vi "HiSPARC Weather Station.vi"() -> ()   [LabVIEW 2012]
uses:
  Globals/Status_Error_Messages.vi
  Globals/Re_Connection_Counter.vi
  Globals/Re_Initialisation_Counter.vi
  Globals/Stop_Data_Loop.vi
  Globals/Stop_Button_Loop.vi
  Globals/USB_WeatherLink_Serialnumber.vi
  Globals/Help_URL.vi
  Globals/DAQ_Mode.vi
  <vilib>/Utility/config.llb/Read Key (Double).vi
  <vilib>/Utility/config.llb/Read Key (Boolean).vi
  <vilib>/Utility/config.llb/Read Key (String).vi
  <vilib>/Utility/config.llb/Read Key (I32).vi
  Globals/TempHumWindDir_Calibration.vi
  Globals/Barometer_Calibration.vi
  Globals/Station_Coordinates.vi
  <vilib>/Platform/browser.llb/Open URL in Default Browser (string).vi
  <vilib>/Utility/config.llb/Write Key (I32).vi
  Globals/PCtime_Last_Data.vi
  <vilib>/Utility/config.llb/Write Key (Boolean).vi
  <vilib>/Utility/config.llb/Write Key (String).vi
  <vilib>/Utility/config.llb/NI_LVConfig.lvlib
  VantagePro.dll
panel:
  in  "Help?":bool
  in  "Stop program?":bool
  in  "DAQ mode?":bool
  out "DAQ software version":string
  in  "Tab Control":T1(tab)
  out "Wind speed [m/s]":dbl(knob)=nan scale=0.0..50.0 scale format="%#.1f"
  out "Forecast":string
  out "Start-time data taking":timestamp=timestamp(-9593251200 s since 1904-01-01) caption="GPS time last data:" format="%< %d/%m/%Y %H:%M>T"
  out "Heat index [°C]":dbl(slide)=nan scale=-20.0..50.0
  out "Solar radiation [W/m²]":dbl(knob)=nan scale=0.0..1500.0
  out "UV index":dbl(knob)=nan scale=0.0..15.0 scale format="%#.1f"
  out "UV High":dbl=nan format="%.1f"
  out "UV Low":dbl=nan format="%.1f"
  out "Solar High":dbl=nan
  out "Solar Low":dbl=nan
  out "Wind direction [º]":dbl(knob)=nan scale=0.0..8.0
  out "Wind High":dbl=nan format="%.1f"
  out "Wind Low":dbl=nan format="%.1f"
  out "Hum out [%]":dbl(slide)=nan caption="Humidity [%]" scale=0.0..100.0 scale format="%#.0f"
  out "Evapotranspiration":dbl(slide)=nan caption="Evapotr. rate [mm/hr]" scale=0.0..50.0 scale format="%#.2f"
  out "Rain rate":dbl(slide)=nan caption="Rain rate [mm/hr]" scale=0.0..50.0 scale format="%#.2f"
  out "Hum. out High":dbl=nan
  out "Hum. out Low":dbl=nan
  out "Evap. High":dbl=nan format="%.2f"
  out "Evap. Low":dbl=nan format="%.2f"
  out "Rain High":dbl=nan format="%.2f"
  out "Rain Low":dbl=nan format="%.2f"
  out "Dew":dbl=nan format="%.1f"
  out "Dew High":dbl=nan format="%.1f"
  out "Dew Low":dbl=nan format="%.1f"
  out "Chill":dbl=nan format="%.1f"
  out "Chill High":dbl=nan format="%.1f"
  out "Chill Low":dbl=nan format="%.1f"
  out "Temp. out":dbl=nan format="%.1f"
  out "Temp. out High":dbl=nan format="%.1f"
  out "Temp. out Low":dbl=nan format="%.1f"
  out "Dew point":dbl(slide)=nan caption="Dew point [°C]" scale=-20.0..50.0
  out "Wind chill [°C]":dbl(slide)=nan scale=-20.0..50.0
  out "Temp out [°C]":dbl(slide)=nan caption="Temperature [°C]" scale=-20.0..50.0
  out "Barometer [hPa]":dbl(slide)=nan scale=940.0..1060.0 scale format="%#.1f"
  out "Hum in [%]":dbl(slide)=nan caption="Humidity [%]" scale=0.0..100.0 scale format="%#.0f"
  out "Temp in [°C]":dbl(slide)=nan caption="Temperature [°C]" scale=-20.0..50.0
  out "Temp. in":dbl=nan format="%.1f"
  out "Temp. in High":dbl=nan format="%.1f"
  out "Temp. in Low":dbl=nan format="%.1f"
  out "Bar. High":dbl=nan format="%.1f"
  out "Bar. Low":dbl=nan format="%.1f"
  out "Hum. in High":dbl=nan
  out "Hum. in Low":dbl=nan
  out "Wind (1h)":cluster{dbl[], dbl[]}[](graph) caption="Wind [1h]"
  out "Evap & heat (1h])":cluster{dbl[], dbl[]}[](graph) caption="Evap & heat [1h]"
  out "Solar radiation (1h)":cluster{dbl[], dbl[]}(graph)
  out "Temperatures (1h)":cluster{dbl[], dbl[]}[](graph) caption="Temperatures [1h]"
  out "Barometer (1h)":cluster{dbl[], dbl[]}(graph)
  out "Humidities (1h)":cluster{dbl[], dbl[]}[](graph)
  out "UV (1h)":cluster{dbl[], dbl[]}(graph)
  out "Wind chill (1h)":cluster{dbl[], dbl[]}(graph)
  out "Rain & dew (1h)":cluster{dbl[], dbl[]}[](graph) caption="Rain & dew [1h]"
  out "Wind (48h)":cluster{dbl[], dbl[]}[](graph) caption="Wind [1h]"
  out "Evap & heat (48h])":cluster{dbl[], dbl[]}[](graph) caption="Evap & heat [1h]"
  out "Solar radiation (48h)":cluster{dbl[], dbl[]}(graph) caption="Solar radiation (1h)"
  out "UV (48h)":cluster{dbl[], dbl[]}(graph) caption="UV (1h)"
  out "Wind chill (48h)":cluster{dbl[], dbl[]}(graph) caption="Wind chill (1h)"
  out "Rain & dew (48h)":cluster{dbl[], dbl[]}[](graph) caption="Rain & dew [1h]"
  out "Temperatures (48h)":cluster{dbl[], dbl[]}[](graph) caption="Temperatures [1h]"
  out "Barometer (48h)":cluster{dbl[], dbl[]}(graph) caption="Barometer (1h)"
  out "Humidities (48h)":cluster{dbl[], dbl[]}[](graph) caption="Humidities (1h)"
  out "GPS time last data":timestamp=timestamp(-9593251200 s since 1904-01-01) caption="GPS time last data:" format="%<%H:%M:%S\n%d/%m/%Y>T"
  out "GPS time correction":i32 caption="GPS time correction [s]:"
  out "Weather station connected?":bool
  out "Run-time error":bool=TRUE
  out "PC time =\nConsole time?":bool caption="PC time = Console time?"
  out "Buffer connected?":bool
  out "Evapotranspiration":u32(colorbox)=7171459
  out "Heat index":u32(colorbox)=7171459
  out "Dew point":u32(colorbox)=7171459
  out "Wind chill":u32(colorbox)=7171459
  out "Temperature":u32(colorbox)=7171459
  out "Rain":u32(colorbox)=7171459
  out "Humidity":u32(colorbox)=7171459
  out "Wind direction":u32(colorbox)=7171459
  out "Wind speed":u32(colorbox)=7171459
  out "Solar radiation":u32(colorbox)=7171459
  out "UV index":u32(colorbox)=7171459
  out "Temperature":u32(colorbox)=7171459
  out "Humidity":u32(colorbox)=7171459
  out "Barometer":u32(colorbox)=7171459
  out "Status/Error messages":string caption="Status messages & error reports"
  in  "Save calibration?":bool
  out "Cur bar":dbl caption="Curr. barometer [hPa]" format="%.1f"
  in  "Barometer sea level [hPa]":dbl min=0.0 max=1060.0 step=0.1 format="%.1f"
  in  "Elevation [m]":i32 min=0 max=500 step=1 format="%#.0f"
  in  "Latitude [º]":dbl min=-90.0 max=90.0 step=0.1 format="%#_14f"
  in  "Longitude [º]":dbl min=-180.0 max=180.0 step=0.1 format="%#.14f"
  out "Cur wind dir":dbl caption="Curr. wind dir. [º]"
  in  "Offset wind dir. [º]":i32 min=-360 max=360 step=1
  out "Cur out hum":dbl caption="Curr. outside hum. [%]" format="%#.0f"
  out "Cur out temp":dbl caption="Curr. outside temp. [°C]" format="%.1f"
  in  "Cal. outside temp. [°C]":dbl min=-40.0 max=65.0 step=0.1 format="%.1f"
  in  "Cal. outside hum. [%]":dbl min=0.0 max=100.0 step=1.0
  out "Cur in hum":dbl caption="Curr. inside hum. [%]" format="%#.0f"
  out "Cur in temp":dbl caption="Curr. inside temp. [°C]" format="%.1f"
  in  "Cal. inside temp. [°C]":dbl min=-40.0 max=65.0 step=0.1 format="%.1f"
  in  "Cal. inside hum. [%]":dbl min=0.0 max=100.0 step=1.0
  out "USB Weather Link":i32
  out "Firmware creation date":string
  out "Software creation date":string=" "
  out "DAQ software version":string
  out "Firmware version":string
  out "Baud rate":i32
  out "COM port":i32
  in  "Database name":string
  in  "Station ID":i32=1 min=1 step=1 format="%#.0f"
  out "Weather station model":string
  out "DLL Version":sgl format="%#.6p"
  in  "Wind chill":bool
  in  "Dew point":bool
  in  "Heat index":bool
  in  "Humidity inside":bool
  in  "Humidity outside":bool
  in  "Rain rate":bool
  in  "Evapotransipration rate":bool
  in  "UV index":bool
  in  "Solar radiation":bool
  in  "Wind speed":bool
  in  "Wind direction":bool
  in  "Barometer":bool
  in  "Temperature outside":bool
  in  "Temperature inside":bool
  in  "Reset settings?":bool
  in  "Save settings?":bool
  in  "Start in DAQ mode?":bool
  # "Inside sensors"
  # "Outside sensors"
  # "Current"
  # "Current"
  # "Low"
  # "Low"
  # "High"
  # "High"
  # "Current"
  # "Low"
  # "High"
  # "Weather forecast, data since"
  # "Low"
  # "Low"
  # "Current"
  # "Current"
  # "High"
  # "High"
  # "Wind direction [°]"
  # "N"
  # "NW"
  # "W"
  # "SW"
  # "S"
  # "SE"
  # "E"
  # "NE"
  # "N"
  # "Wind direction [°]"
  # "N"
  # "NW"
  # "W"
  # "SW"
  # "S"
  # "SE"
  # "E"
  # "NE"
  # "N"
  # "Status station"
  # "Status derived properties"
  # "Status outside sensors"
  # "Status inside sensors"
  # "Calibration parameters"
  # "General station parameters"
  # "Sensor selection"
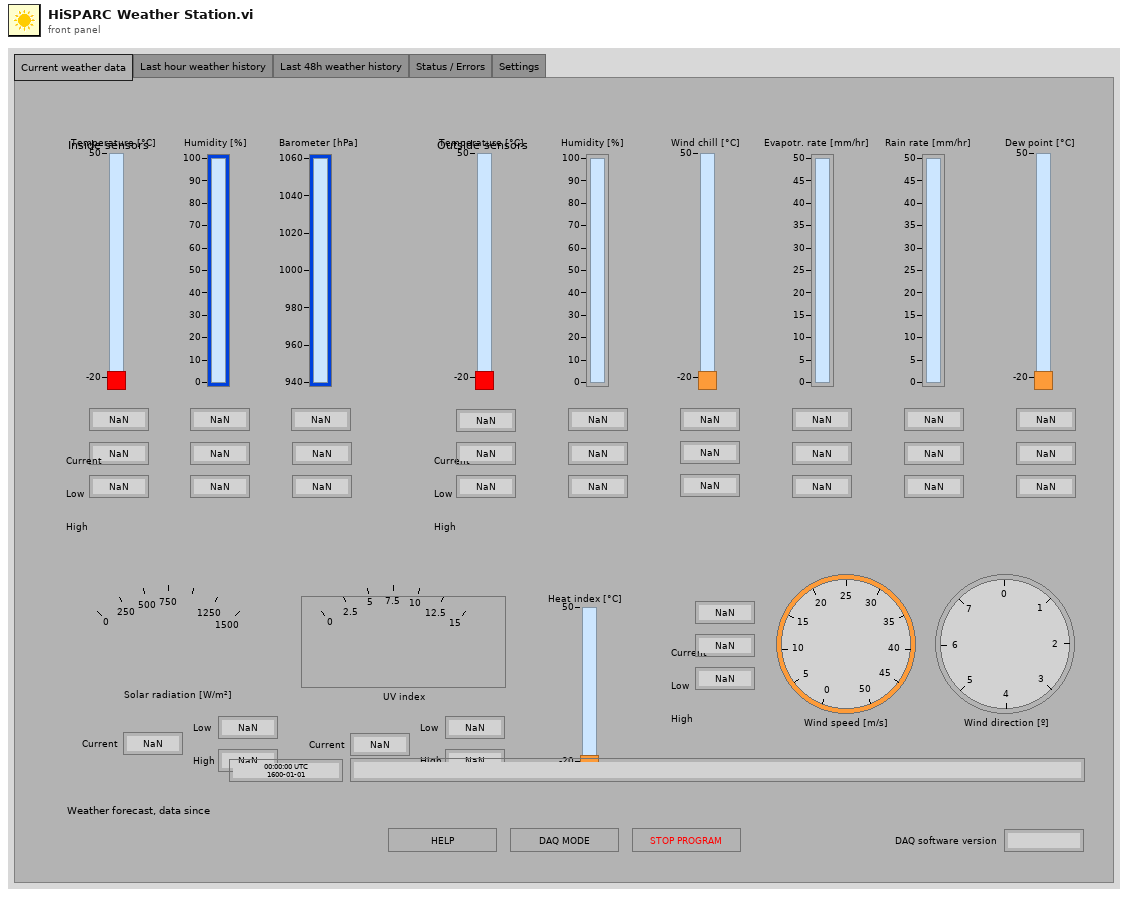
[diagram p1: front panel]
types:
  T1 = enum32{"Current weather data", "Last hour weather history", "Last 48h weather history", "Status / Errors", "Settings"}
  T2 = cluster{"Path Run Status file":path, "Path Default Settings file":path, "Path User Settings file":path}
  T3 = cluster{"Data out":dbl, "Data out":dbl, "Data out":dbl, "Data out":dbl, "Data out":dbl, "Data out":dbl, "Data out":dbl, "Data out":dbl, "Data out":dbl, "Data out":dbl, "Data out":dbl, "Data out":dbl, "Data out":dbl, "Data out":dbl, "seconds since 1Jan1904":dbl}
  T4 = typedef "NI_LVConfig.lvlib/Config Data RefNum.ctl" = refnum<k1>
  T5 = cluster{"TempUnit":i8, "RainUnit":i8, "PressUnit":i8, "WindUnit":i8, "ElevUnit":i8}
  T6 = cluster{"Temperature_inside":sgl, "Temperature_outside":sgl, "Humidity_inside":sgl, "Humidity_outside":sgl, "Barometer":sgl, "Wind_direction":sgl, "Wind_speed":sgl, "Solar_radiation":sgl, "UV_index":sgl, "Evapotranspiration":sgl, "Rain_rate":sgl, "Heat_index":sgl, "Dew_point":sgl, "Wind_chill":sgl}
  T7 = cluster{"Data out":dbl, "Data out":dbl, "Data out":dbl, "Data out":dbl, "Data out":dbl, "Data out":dbl, "Data out":dbl, "Data out":dbl, "Data out":dbl, "Data out":dbl, "Data out":dbl, "Data out":dbl, "Data out":dbl, "Data out":dbl, "seconds since 1Jan1904":dbl}[]
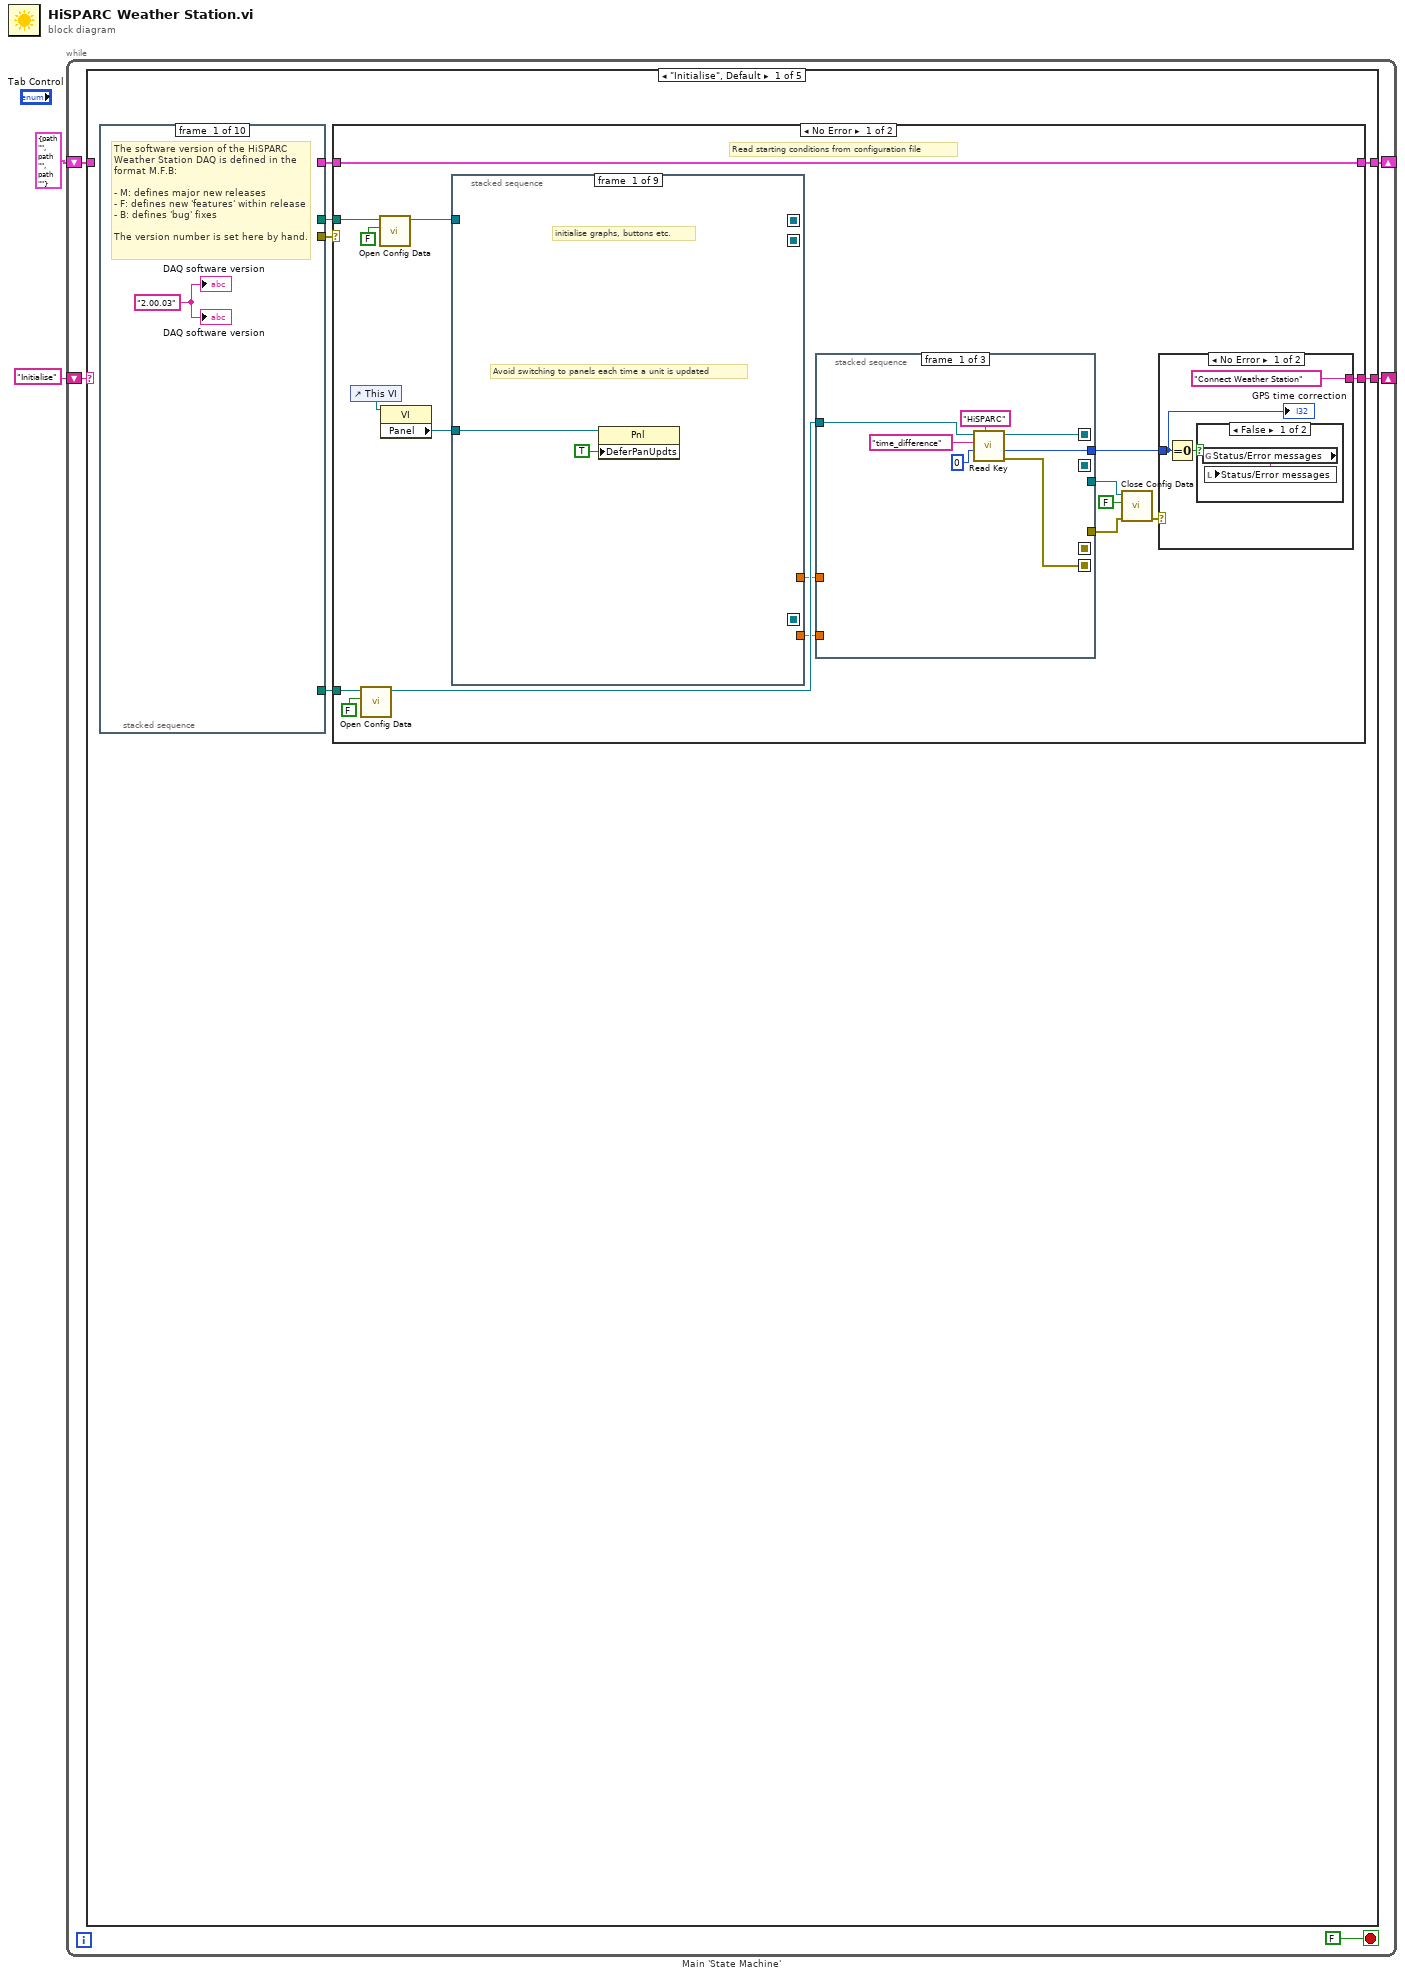
[diagram p0: block diagram]
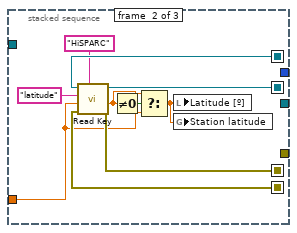
[diagram p2: hidden frame]
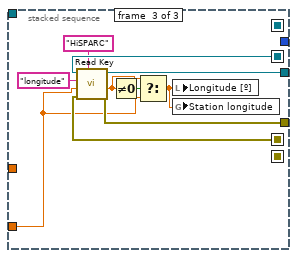
[diagram p3: hidden frame]
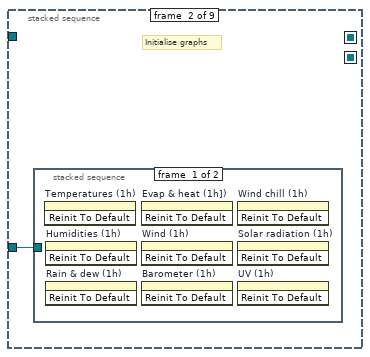
[diagram p4: hidden frame]
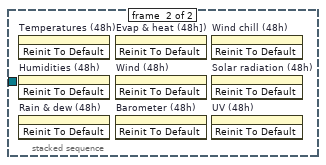
[diagram p5: hidden frame]
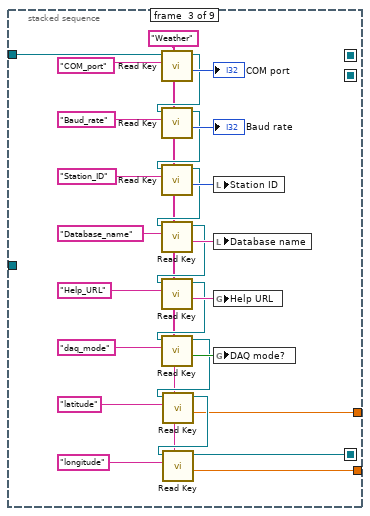
[diagram p6: hidden frame]
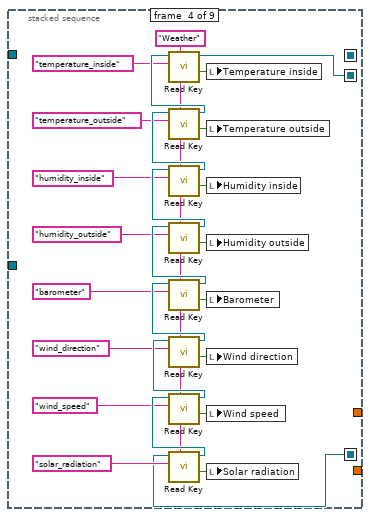
[diagram p7: hidden frame]
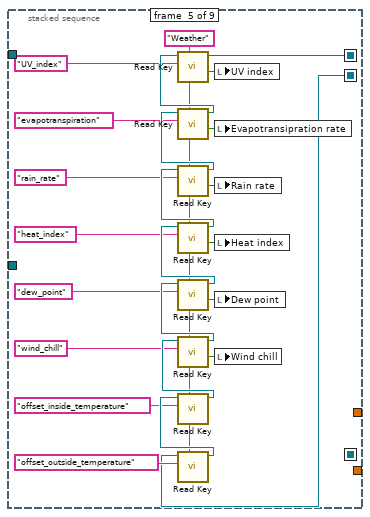
[diagram p8: hidden frame]
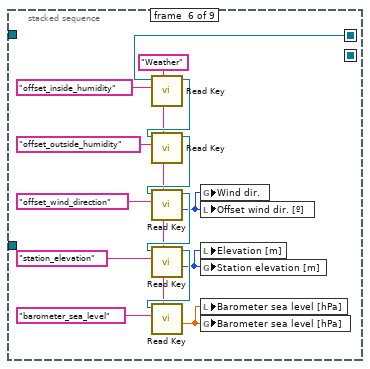
[diagram p9: hidden frame]
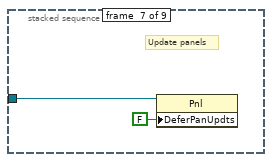
[diagram p10: hidden frame]
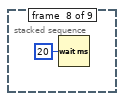
[diagram p11: hidden frame]
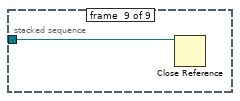
[diagram p12: hidden frame]
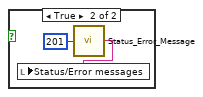
[diagram p13: hidden frame]
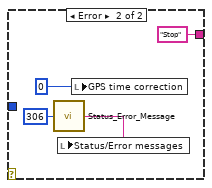
[diagram p14: hidden frame]
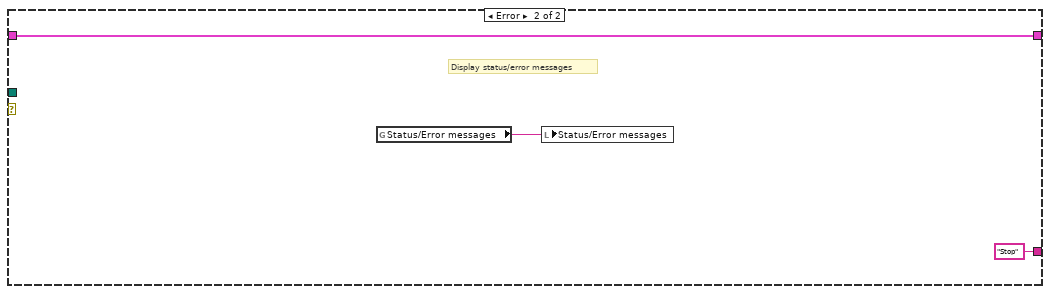
[diagram p15: hidden frame]
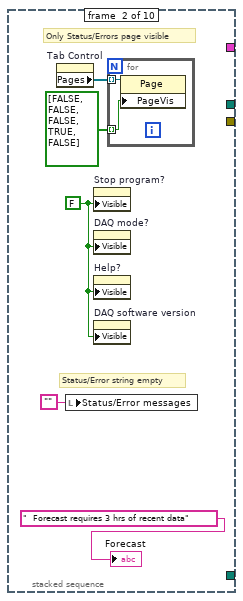
[diagram p16: hidden frame]
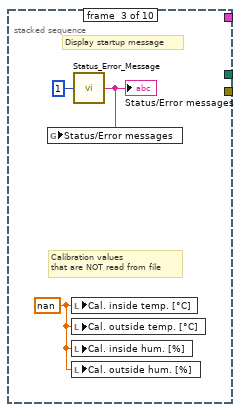
[diagram p17: hidden frame]
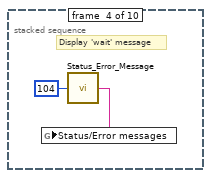
[diagram p18: hidden frame]
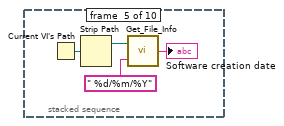
[diagram p19: hidden frame]
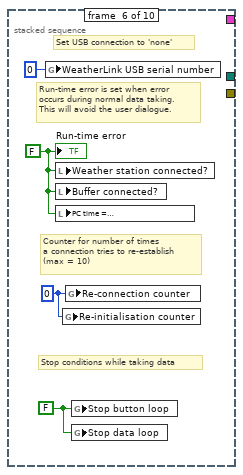
[diagram p20: hidden frame]
diagram:
  n1 = while "Main 'State Machine'" {
    shift-right: [w7] -> _
    shift-left: "Initialise" -> [w4]
    shift-right: [w6] -> _
    shift-left: T2 {"Path Run Status file"=path "", "Path Default Settings file"=path "", "Path User Settings file"=path ""} ("Paths ini files") -> [w5]
    stop <- FALSE stop-if-true
    n2 = case shown="\"Initialise\", Default" w4 {
      selector: w4 -> [_ _ _ _ w1338]
      tunnel: [w12 w222 w371 w535 w1339] -> w7
      tunnel: [w13 w217 w376 w539 w1340] -> w6
      tunnel: w5 -> [_ w223 w376 w530 w1340]
      frame "Initialise", Default {
        n3 = stacked-sequence {
          tunnel: [_ _ _ _ _ _ _ _ _ w210] -> w11
          tunnel: [_ _ _ _ _ _ _ _ _ w212] -> w10
          tunnel: [_ _ _ _ _ _ _ _ _ w211] -> w9
          tunnel: [_ _ _ _ _ _ _ _ _ w209] -> w8
          frame #0 {
            w168 = "2.00.03"
            # "The software version of the HiSPARC\nWeather Station DAQ is defined in the\nformat M.F.B:\n\n- M: defines major new releases\n- F: defines new 'features' within release\n- B: defines 'bug' fixes\n\nThe version number is set here by hand."
            "DAQ software version" <- w168
            "DAQ software version" <- w168
          }
          frame #1 {
            w173 = FALSE ("Visible")
            # "Status/Error string empty"
            # "Only Status/Errors page visible"
            n4 = property on="Tab Control" class="TabCtl (strict)"() -> ("Pages"=w171:refnum<vi>[])  [unwired: 2 in, 2 out]
            n5 = local write "Status/Error messages"("") -> ()
            n6 = property on="Stop program?" class="Bool (strict)"("Visible"=w173) -> ()  [unwired: 2 in, 2 out]
            n7 = property on="DAQ mode?" class="Bool (strict)"("Visible"=w173) -> ()  [unwired: 2 in, 2 out]
            n8 = property on="Help?" class="Bool (strict)"("Visible"=w173) -> ()  [unwired: 2 in, 2 out]
            n9 = property on="DAQ software version" class="Str"("Visible"=w173) -> ()  [unwired: 2 in, 2 out]
            n10 = for {
              tunnel: bool[] [FALSE, FALSE, FALSE, TRUE, FALSE] -> [w175] mode=indexing
              tunnel: w171 -> [w174] mode=indexing
              n11 = property class="Page"(reference=w174, "PageVis"=w175) -> ()  [unwired: 1 in, 2 out]
            }
            "Forecast" <- "  Forecast requires 3 hrs of recent data" ("Forecast")
          }
          frame #2 {
            w176 = nan ("Data_input")
            # "Calibration values\nthat are NOT read from file"
            # "Display startup message"
            n12 = local write "Cal. inside temp. [°C]"(w176) -> ()
            n13 = local write "Cal. outside temp. [°C]"(w176) -> ()
            n14 = local write "Cal. inside hum. [%]"(w176) -> ()
            n15 = local write "Cal. outside hum. [%]"(w176) -> ()
            n16 = call "Status_Error_Message.vi"("Message number"=1) -> ("Status/Error string"=w177:string)
            "Status/Error messages" <- w177
            n17 = global write "Status_Error_Messages.vi" "Status/Error messages"(w177) -> ()
          }
          frame #3 {
            # "Display 'wait' message"
            n18 = call "Status_Error_Message.vi"("Message number"=104) -> ("Status/Error string"=w179:string)
            n19 = global write "Status_Error_Messages.vi" "Status/Error messages"(w179) -> ()
          }
          frame #4 {
            n20 = Current VI's Path() -> (path=w182:path)
            n21 = Strip Path(path=w182) -> (stripped path=w184:path)  [unwired: 1 out]
            n22 = call "Get_File_Info.vi"("Time Format String (%c)"=" %d/%m/%Y", "File Path"=w184) -> ("Creation Date"=→"Software creation date":string)
          }
          frame #5 {
            w185 = FALSE
            w188 = u32 0 ("Re-connection counter")
            w186 = FALSE
            # "Set USB connection to 'none'"
            # "Stop conditions while taking data"
            # "Counter for number of times\na connection tries to re-establish\n(max = 10)"
            # "Run-time error is set when error\noccurs during normal data taking.\nThis will avoid the user dialogue."
            n23 = global write "USB_WeatherLink_Serialnumber.vi" "WeatherLink USB serial number"(u32 0 ("WeatherLink USB serial number")) -> ()
            n24 = local write "Weather station connected?"(w186) -> ()
            n25 = local write "Buffer connected?"(w186) -> ()
            n26 = local write "PC time =\nConsole time?"(w186) -> ()
            n27 = global write "Re_Initialisation_Counter.vi" "Re-initialisation counter"(w188) -> ()
            n28 = global write "Re_Connection_Counter.vi" "Re-connection counter"(w188) -> ()
            n29 = global write "Stop_Button_Loop.vi" "Stop button loop"(w185) -> ()
            n30 = global write "Stop_Data_Loop.vi" "Stop data loop"(w185) -> ()
            "Run-time error" <- w186
          }
          frame #6 {
            # "Initialise data queue"
            n31 = Obtain Queue(max queue size (-1, unlimited)=30, name (unnamed)="Weather data (5 s)", element data type=T3 {"Data out"=0.0, "Data out"=0.0, "Data out"=0.0, "Data out"=0.0, "Data out"=0.0, "Data out"=0.0, "Data out"=0.0, "Data out"=0.0, "Data out"=0.0, "Data out"=0.0, "Data out"=0.0, "Data out"=0.0, "Data out"=0.0, "Data out"=0.0, "seconds since 1Jan1904"=0.0} ("output cluster"), create if not found? (T)=TRUE) -> (queue out=w192:refnum<queue>)  [unwired: 1 in, 2 out]
            n32 = Flush Queue(queue=w192) -> ()  [unwired: 1 in, 3 out]
          }
          frame #7 {
            # "Initialise daytabase queue"
            n33 = Obtain Queue(max queue size (-1, unlimited)=60, name (unnamed)="Database queue", element data type="" ("Weather parameter string"), create if not found? (T)=TRUE) -> (queue out=w197:refnum<queue>)  [unwired: 1 in, 2 out]
            n34 = Flush Queue(queue=w197) -> ()  [unwired: 1 in, 3 out]
          }
          frame #8 {
            # "Initialise graph queues"
            n35 = Obtain Queue(max queue size (-1, unlimited)=61, name (unnamed)="60 minutes data queue", element data type=T3 {"Data out"=0.0, "Data out"=0.0, "Data out"=0.0, "Data out"=0.0, "Data out"=0.0, "Data out"=0.0, "Data out"=0.0, "Data out"=0.0, "Data out"=0.0, "Data out"=0.0, "Data out"=0.0, "Data out"=0.0, "Data out"=0.0, "Data out"=0.0, "seconds since 1Jan1904"=0.0} ("output cluster"), create if not found? (T)=TRUE) -> (queue out=w207:refnum<queue>)  [unwired: 1 in, 2 out]
            n36 = Obtain Queue(max queue size (-1, unlimited)=289, name (unnamed)="48 hours data queue", element data type=T3 {"Data out"=0.0, "Data out"=0.0, "Data out"=0.0, "Data out"=0.0, "Data out"=0.0, "Data out"=0.0, "Data out"=0.0, "Data out"=0.0, "Data out"=0.0, "Data out"=0.0, "Data out"=0.0, "Data out"=0.0, "Data out"=0.0, "Data out"=0.0, "seconds since 1Jan1904"=0.0} ("output cluster"), create if not found? (T)=TRUE) -> (queue out=w202:refnum<queue>)  [unwired: 1 in, 2 out]
            n37 = Flush Queue(queue=w207) -> ()  [unwired: 1 in, 3 out]
            n38 = Flush Queue(queue=w202) -> ()  [unwired: 1 in, 3 out]
          }
          frame #9 {
            # "Determine paths configuration files"
            n39 = call "Get_Ini_File_Paths.vi"() -> ("Error out"=w211:errorcluster, "Paths ini files"=w210:T2)  [unwired: 2 in]
            n40 = Unbundle By Name(w210) -> ("Path User Settings file"=w212:path)
            n41 = Unbundle By Name(w210) -> ("Path Run Status file"=w209:path)
          }
        }
        n42 = case shown="No Error" w9 {
          tunnel: w10 -> [w25 _]
          tunnel: w11 -> [w26 w166]
          tunnel: [w27 "Stop"] -> w12
          tunnel: [w26 w166] -> w13
          tunnel: w8 -> [w23 _]
          frame No Error {
            # "Read starting conditions from configuration file"
            n43 = control-ref of="This VI"() -> (w15:refnum<vi>)
            n44 = call <vilib>:"Open Config Data.vi"("create file if necessary (T)"=FALSE, "configuration file path"=w23) -> ("refnum"=w21:T4)  [unwired: 7 in, 2 out]
            n45 = call <vilib>:"Open Config Data.vi"("create file if necessary (T)"=FALSE, "configuration file path"=w25) -> ("refnum"=w22:T4)  [unwired: 7 in, 2 out]
            n46 = property class="VI"(reference=w15) -> ("Panel"=w14:refnum<vi>)  [unwired: 1 in, 2 out]
            n47 = stacked-sequence {
              seq-local: [_ _ w62 _ _ _ _ _ _] -> [_ _ _ w89 _ _ _ _ _]
              seq-local: [_ _ _ w88 _ _ _ _ _] -> [_ _ _ _ w115 _ _ _ _]
              seq-local: [_ _ _ _ w114 _ _ _ _] -> [_ _ _ _ _ w141 _ _ _]
              tunnel: w22 -> [_ _ w74 _ _ _ _ _ _]
              tunnel: [_ _ w71 _ _ _ _ _ _] -> w16
              tunnel: [_ _ w63 _ _ _ _ _ _] -> w17
              tunnel: w14 -> [w58 w60 _ _ _ _ w151 _ w154]
              frame #0 {
                # "Avoid switching to panels each time a unit is updated"
                # "initialise graphs, buttons etc."
                n48 = property class="Pnl"(reference=w58, "DeferPanUpdts"=TRUE ("Defer Panel Updates")) -> ()  [unwired: 1 in, 2 out]
              }
              frame #1 {
                # "Initialise graphs"
                n49 = stacked-sequence {
                  tunnel: w60 -> [_ _]
                  frame #0 {
                    n50 = invoke on="Temperatures (1h)" class="XYGraph (strict)" method="Reinit To Default"() -> ()  [unwired: 3 in, 3 out]
                    n51 = invoke on="Humidities (1h)" class="XYGraph (strict)" method="Reinit To Default"() -> ()  [unwired: 3 in, 3 out]
                    n52 = invoke on="Rain & dew (1h)" class="XYGraph (strict)" method="Reinit To Default"() -> ()  [unwired: 3 in, 3 out]
                    n53 = invoke on="Evap & heat (1h])" class="XYGraph (strict)" method="Reinit To Default"() -> ()  [unwired: 3 in, 3 out]
                    n54 = invoke on="Wind (1h)" class="XYGraph (strict)" method="Reinit To Default"() -> ()  [unwired: 3 in, 3 out]
                    n55 = invoke on="Barometer (1h)" class="XYGraph (strict)" method="Reinit To Default"() -> ()  [unwired: 3 in, 3 out]
                    n56 = invoke on="Wind chill (1h)" class="XYGraph (strict)" method="Reinit To Default"() -> ()  [unwired: 3 in, 3 out]
                    n57 = invoke on="Solar radiation (1h)" class="XYGraph (strict)" method="Reinit To Default"() -> ()  [unwired: 3 in, 3 out]
                    n58 = invoke on="UV (1h)" class="XYGraph (strict)" method="Reinit To Default"() -> ()  [unwired: 3 in, 3 out]
                  }
                  frame #1 {
                    n59 = invoke on="Temperatures (48h)" class="XYGraph (strict)" method="Reinit To Default"() -> ()  [unwired: 3 in, 3 out]
                    n60 = invoke on="Humidities (48h)" class="XYGraph (strict)" method="Reinit To Default"() -> ()  [unwired: 3 in, 3 out]
                    n61 = invoke on="Rain & dew (48h)" class="XYGraph (strict)" method="Reinit To Default"() -> ()  [unwired: 3 in, 3 out]
                    n62 = invoke on="Evap & heat (48h])" class="XYGraph (strict)" method="Reinit To Default"() -> ()  [unwired: 3 in, 3 out]
                    n63 = invoke on="Wind (48h)" class="XYGraph (strict)" method="Reinit To Default"() -> ()  [unwired: 3 in, 3 out]
                    n64 = invoke on="Barometer (48h)" class="XYGraph (strict)" method="Reinit To Default"() -> ()  [unwired: 3 in, 3 out]
                    n65 = invoke on="Wind chill (48h)" class="XYGraph (strict)" method="Reinit To Default"() -> ()  [unwired: 3 in, 3 out]
                    n66 = invoke on="Solar radiation (48h)" class="XYGraph (strict)" method="Reinit To Default"() -> ()  [unwired: 3 in, 3 out]
                    n67 = invoke on="UV (48h)" class="XYGraph (strict)" method="Reinit To Default"() -> ()  [unwired: 3 in, 3 out]
                  }
                }
              }
              frame #2 {
                w61 = "Weather" ("section")
                n68 = call-poly <vilib>:"Read Key.vi"("section"=w61, "key"="COM_port", "refnum"=w74) -> ("value"=→"COM port":i32, "refnum out"=w73:T4)  [unwired: 5 in, 2 out]
                n69 = call-poly <vilib>:"Read Key.vi"("section"=w61, "key"="Baud_rate", "refnum"=w73) -> ("value"=→"Baud rate":i32, "refnum out"=w72:T4)  [unwired: 5 in, 2 out]
                n70 = call-poly <vilib>:"Read Key.vi"("section"=w61, "key"="Station_ID", "refnum"=w72) -> ("value"=w84:i32, "refnum out"=w68:T4)  [unwired: 5 in, 2 out]
                n71 = call-poly <vilib>:"Read Key.vi"("section"=w61, "key"="Database_name" ("Key name"), "refnum"=w68) -> ("value"=w83:string, "refnum out"=w67:T4)  [unwired: 5 in, 2 out]
                n72 = call-poly <vilib>:"Read Key.vi"("section"=w61, "key"="Help_URL" ("Key name"), "refnum"=w67) -> ("value"=w82:string, "refnum out"=w66:T4)  [unwired: 5 in, 2 out]
                n73 = call-poly <vilib>:"Read Key.vi"("section"=w61, "key"="daq_mode", "refnum"=w66) -> ("value"=w81:bool, "refnum out"=w65:T4)  [unwired: 5 in, 2 out]
                n74 = call-poly <vilib>:"Read Key.vi"("section"=w61, "key"="latitude", "refnum"=w65) -> ("value"=w63:dbl, "refnum out"=w64:T4)  [unwired: 5 in, 2 out]
                n75 = call-poly <vilib>:"Read Key.vi"("section"=w61, "key"="longitude", "refnum"=w64) -> ("value"=w71:dbl, "refnum out"=w62:T4)  [unwired: 5 in, 2 out]
                n76 = local write "Station ID"(w84) -> ()
                n77 = local write "Database name"(w83) -> ()
                n78 = global write "Help_URL.vi" "Help URL"(w82) -> ()
                n79 = global write "DAQ_Mode.vi" "DAQ mode?"(w81) -> ()
              }
              frame #3 {
                w87 = "Weather" ("section")
                n80 = call-poly <vilib>:"Read Key.vi"("section"=w87, "key"="solar_radiation", "refnum"=w89) -> ("value"=w105:bool, "refnum out"=w106:T4)  [unwired: 5 in, 2 out]
                n81 = call-poly <vilib>:"Read Key.vi"("section"=w87, "key"="wind_speed", "refnum"=w106) -> ("value"=w104:bool, "refnum out"=w111:T4)  [unwired: 5 in, 2 out]
                n82 = call-poly <vilib>:"Read Key.vi"("section"=w87, "key"="wind_direction", "refnum"=w111) -> ("value"=w103:bool, "refnum out"=w112:T4)  [unwired: 5 in, 2 out]
                n83 = call-poly <vilib>:"Read Key.vi"("section"=w87, "key"="barometer", "refnum"=w112) -> ("value"=w102:bool, "refnum out"=w107:T4)  [unwired: 5 in, 2 out]
                n84 = call-poly <vilib>:"Read Key.vi"("section"=w87, "key"="humidity_outside", "refnum"=w107) -> ("value"=w101:bool, "refnum out"=w108:T4)  [unwired: 5 in, 2 out]
                n85 = call-poly <vilib>:"Read Key.vi"("section"=w87, "key"="humidity_inside", "refnum"=w108) -> ("value"=w90:bool, "refnum out"=w109:T4)  [unwired: 5 in, 2 out]
                n86 = call-poly <vilib>:"Read Key.vi"("section"=w87, "key"="temperature_outside", "refnum"=w109) -> ("value"=w91:bool, "refnum out"=w110:T4)  [unwired: 5 in, 2 out]
                n87 = call-poly <vilib>:"Read Key.vi"("section"=w87, "key"="temperature_inside", "refnum"=w110) -> ("value"=w92:bool, "refnum out"=w88:T4)  [unwired: 5 in, 2 out]
                n88 = local write "Temperature inside"(w92) -> ()
                n89 = local write "Temperature outside"(w91) -> ()
                n90 = local write "Humidity inside"(w90) -> ()
                n91 = local write "Humidity outside"(w101) -> ()
                n92 = local write "Barometer"(w102) -> ()
                n93 = local write "Wind direction"(w103) -> ()
                n94 = local write "Wind speed"(w104) -> ()
                n95 = local write "Solar radiation"(w105) -> ()
              }
              frame #4 {
                w113 = "Weather" ("section")
                n96 = call-poly <vilib>:"Read Key.vi"("section"=w113, "key"="offset_outside_temperature", "refnum"=w115) -> ("refnum out"=w130:T4)  [unwired: 5 in, 3 out]
                n97 = call-poly <vilib>:"Read Key.vi"("section"=w113, "key"="offset_inside_temperature", "refnum"=w130) -> ("refnum out"=w135:T4)  [unwired: 5 in, 3 out]
                n98 = call-poly <vilib>:"Read Key.vi"("section"=w113, "key"="wind_chill", "refnum"=w135) -> ("value"=w120:bool, "refnum out"=w136:T4)  [unwired: 5 in, 2 out]
                n99 = call-poly <vilib>:"Read Key.vi"("section"=w113, "key"="dew_point", "refnum"=w136) -> ("value"=w116:bool, "refnum out"=w131:T4)  [unwired: 5 in, 2 out]
                n100 = call-poly <vilib>:"Read Key.vi"("section"=w113, "key"="heat_index", "refnum"=w131) -> ("value"=w117:bool, "refnum out"=w132:T4)  [unwired: 5 in, 2 out]
                n101 = call-poly <vilib>:"Read Key.vi"("section"=w113, "key"="rain_rate", "refnum"=w132) -> ("value"=w118:bool, "refnum out"=w133:T4)  [unwired: 5 in, 2 out]
                n102 = call-poly <vilib>:"Read Key.vi"("section"=w113, "key"="evapotranspiration", "refnum"=w133) -> ("value"=w119:bool, "refnum out"=w134:T4)  [unwired: 5 in, 2 out]
                n103 = call-poly <vilib>:"Read Key.vi"("section"=w113, "key"="UV_index", "refnum"=w134) -> ("value"=w121:bool, "refnum out"=w114:T4)  [unwired: 5 in, 2 out]
                n104 = local write "UV index"(w121) -> ()
                n105 = local write "Evapotransipration rate"(w119) -> ()
                n106 = local write "Rain rate"(w118) -> ()
                n107 = local write "Heat index"(w117) -> ()
                n108 = local write "Dew point"(w116) -> ()
                n109 = local write "Wind chill"(w120) -> ()
              }
              frame #5 {
                w137 = "Weather" ("section")
                n110 = call-poly <vilib>:"Read Key.vi"("section"=w137, "key"="offset_inside_humidity", "refnum"=w141) -> ("refnum out"=w150:T4)  [unwired: 5 in, 3 out]
                n111 = call-poly <vilib>:"Read Key.vi"("section"=w137, "key"="offset_outside_humidity", "refnum"=w150) -> ("refnum out"=w149:T4)  [unwired: 5 in, 3 out]
                n112 = call-poly <vilib>:"Read Key.vi"("section"=w137, "key"="offset_wind_direction", "refnum"=w149) -> ("value"=w140:i32, "refnum out"=w148:T4)  [unwired: 5 in, 2 out]
                n113 = call-poly <vilib>:"Read Key.vi"("section"=w137, "key"="station_elevation", "refnum"=w148) -> ("value"=w139:i32, "refnum out"=w147:T4)  [unwired: 5 in, 2 out]
                n114 = call-poly <vilib>:"Read Key.vi"("section"=w137, "key"="barometer_sea_level", "refnum"=w147) -> ("value"=w138:dbl)  [unwired: 5 in, 3 out]
                n115 = global write "TempHumWindDir_Calibration.vi" "Wind dir."(w140) -> ()
                n116 = local write "Offset wind dir. [º]"(w140) -> ()
                n117 = local write "Elevation [m]"(w139) -> ()
                n118 = global write "Barometer_Calibration.vi" "Station elevation [m]"(w139) -> ()
                n119 = local write "Barometer sea level [hPa]"(w138) -> ()
                n120 = global write "Barometer_Calibration.vi" "Barometer sea level [hPa]"(w138) -> ()
              }
              frame #6 {
                # "Update panels"
                n121 = property class="Pnl"(reference=w151, "DeferPanUpdts"=FALSE ("Defer Panel Updates")) -> ()  [unwired: 1 in, 2 out]
              }
              frame #7 {
                n122 = Wait (ms)(milliseconds to wait=u32 20) -> ()  [unwired: 1 out]
              }
              frame #8 {
                n123 = Close Reference(reference=w154) -> ()  [unwired: 1 in, 1 out]
              }
            }
            n124 = stacked-sequence {
              seq-local: [w34 _ _] -> [_ w43 _]
              seq-local: [_ w42 _] -> [_ _ w53]
              seq-local: [w33 _ _] -> [_ w41 _]
              seq-local: [_ w40 _] -> [_ _ w51]
              tunnel: w21 -> [w35 _ _]
              tunnel: [_ _ w52] -> w19
              tunnel: [w32 _ _] -> w18
              tunnel: [_ _ w50] -> w20
              tunnel: w17 -> [_ w39 _]
              tunnel: w16 -> [_ _ w49]
              frame #0 {
                n125 = call-poly <vilib>:"Read Key.vi"("section"="HiSPARC", "default value"=0, "key"="time_difference", "refnum"=w35) -> ("error out"=w33:errorcluster, "value"=w32:i32, "refnum out"=w34:T4)  [unwired: 4 in, 1 out]
              }
              frame #1 {
                n126 = call-poly <vilib>:"Read Key.vi"("section"="HiSPARC", "error in (no error)"=w41, "default value"=w39, "key"="latitude", "refnum"=w43) -> ("error out"=w40:errorcluster, "value"=w46:dbl, "refnum out"=w42:T4)  [unwired: 3 in, 1 out]
                n127 = Not Equal To 0?(x=w46) -> (x != 0?=w45:bool)
                n128 = Select(t=w46, s=w45, f=w39) -> (s? t:f=w47:dbl)
                n129 = local write "Latitude [º]"(w47) -> ()
                n130 = global write "Station_Coordinates.vi" "Station latitude"(w47) -> ()
              }
              frame #2 {
                n131 = call-poly <vilib>:"Read Key.vi"("section"="HiSPARC", "error in (no error)"=w51, "default value"=w49, "key"="longitude", "refnum"=w53) -> ("error out"=w52:errorcluster, "value"=w56:dbl, "refnum out"=w50:T4)  [unwired: 3 in, 1 out]
                n132 = Not Equal To 0?(x=w56) -> (x != 0?=w55:bool)
                n133 = Select(t=w56, s=w55, f=w49) -> (s? t:f=w57:dbl)
                n134 = local write "Longitude [º]"(w57) -> ()
                n135 = global write "Station_Coordinates.vi" "Station longitude"(w57) -> ()
              }
            }
            n136 = call <vilib>:"Close Config Data.vi"("error in (no error)"=w19, "write file if changed (T)"=FALSE, "refnum"=w20) -> ("error out"=w28:errorcluster)  [unwired: 7 in, 1 out]
            n137 = case shown="No Error" w28 {
              tunnel: ["Connect Weather Station" "Stop"] -> w27
              tunnel: w18 -> [w157 _]
              frame No Error {
                n138 = Equal To 0?(x=w157) -> (x = 0?=w156:bool)
                n139 = case shown="False" w156 {
                  frame False {
                    n140 = global read "Status_Error_Messages.vi" "Status/Error messages"() -> (w158:string)
                    n141 = local write "Status/Error messages"(w158) -> ()
                  }
                  frame True {
                    n142 = call "Status_Error_Message.vi"("Message number"=201) -> ("Status/Error string"=w159:string)
                    n143 = local write "Status/Error messages"(w159) -> ()
                  }
                }
                "GPS time correction" <- w157
              }
              frame Error {
                n144 = call "Status_Error_Message.vi"("Message number"=306) -> ("Status/Error string"=w162:string)
                n145 = local write "Status/Error messages"(w162) -> ()
                n146 = local write "GPS time correction"(0 ("GPS time correction")) -> ()
              }
            }
          }
          frame Error {
            # "Display status/error messages"
            n147 = global read "Status_Error_Messages.vi" "Status/Error messages"() -> (w165:string)
            n148 = local write "Status/Error messages"(w165) -> ()
          }
        }
      }
      frame "Connect Weather Station" {
        w213 = u32 7171459
        # "Please select:\n\n- COM port number\n  - Launch the Windows 'Device Manager' (Apparatenbeheer)\n  - Open 'COM & LPT'\n  - Windows assigned a 'COM number' for your serial connection\n\n- Baud rate\n  - Speed at which your weather station communicates with your computer\n  - Default: 19200\n\n- Station ID\n  - Iidentifier for your station distributed together with your certificate\n    (required during software installation)\n  - Usually the same ID as your cosmic ray detector\n  - The ID of your cosmic ray station is stored in: Z:\\ persistent\\config.ini"
        # "Connect weather station"
        n149 = local read "COM port"() -> (w219:i32)
        n150 = local read "Baud rate"() -> (w220:i32)
        n151 = local read "Station ID"() -> (w221:i32)
        n152 = local read "Run-time error"() -> (w215:bool)
        n153 = call "Open_WeatherStation_Connection.vi"("Station ID"=w221, "Baud rate"=w220, "COM port"=w219) -> ("Weather station connected?"=w214:bool)
        n154 = Or(x=w214, y=w215) -> (x .or. y?=w216:bool)
        n155 = case shown="False" w216 {
          selector: w216 -> [w230 w337]
          tunnel: w221 -> [w238 _]
          tunnel: w220 -> [w239 _]
          tunnel: w219 -> [w240 _]
          tunnel: w223 -> [w233 w340]
          tunnel: [w231 w339] -> w222
          tunnel: [w230 w336] -> w218
          tunnel: [w229 w340] -> w217
          tunnel: w214 -> [_ w338]
          frame False {
            n156 = flat-sequence {
              tunnel: w233 -> [w242]
              tunnel: w238 -> [w243]
              tunnel: w239 -> [w244]
              tunnel: w240 -> [w245]
              tunnel: [w245] -> w228
              tunnel: [w244] -> w227
              tunnel: [w243] -> w226
              tunnel: [w242] -> w225
              tunnel: [w253] -> w237
              tunnel: [w252] -> w236
              tunnel: [w251] -> w235
              tunnel: [w250] -> w234
              tunnel: [w249] -> w232
              tunnel: w228 -> [w256]
              tunnel: w227 -> [w255]
              tunnel: w226 -> [w254]
              tunnel: w225 -> [w249]
              tunnel: [w247] -> w224
              tunnel: w237 -> [w283]
              tunnel: w236 -> [w282]
              tunnel: w235 -> [w281]
              tunnel: w234 -> [w280]
              tunnel: w232 -> [w279]
              tunnel: [w275] -> w231
              tunnel: [w274] -> w229
              tunnel: w224 -> [w273]
              frame #0 {
                # "Hide all tabs"
                n157 = property on="Tab Control" class="TabCtl (strict)"("Visible"=FALSE) -> ()  [unwired: 2 in, 2 out]
              }
              frame #1 {
                # "Warn user!"
                n158 = global read "USB_WeatherLink_Serialnumber.vi" "WeatherLink USB serial number"() -> (w246:u32)
                n159 = call <vilib>:"Beep.vi"("use system alert? (T)"=TRUE) -> ()  [unwired: 11 in]
                n160 = case shown="1, Default" w246 {
                  tunnel: w256 -> [w264 w268]
                  tunnel: w255 -> [w263 w269]
                  tunnel: w254 -> [w262 w271]
                  tunnel: [w261 w266] -> w253
                  tunnel: [w260 w265] -> w252
                  tunnel: [w259 w267] -> w251
                  tunnel: [w258 w270] -> w250
                  tunnel: [w257 w272] -> w247
                  frame 0 {
                    n161 = call "Station_Port_Dialog_Serial.vi"("Station ID in"=w262, "Baud rate in"=w263, "COM port in"=w264) -> ("Station ID out"=w258:i32, "Baud rate out"=w261:i32, "COM port out"=w259:i32, "OK"=w260:bool, "Help?"=w257:bool)  [unwired: 2 in, 1 out]
                  }
                  frame 1, Default {
                    n162 = call "Station_Port_Dialog_USB.vi"("Station ID in"=w271, "Baud rate in"=w269, "COM port in"=w268) -> ("Station ID out"=w270:i32, "Baud rate out"=w266:i32, "COM port out"=w267:i32, "OK"=w265:bool, "Help?"=w272:bool)  [unwired: 2 in, 1 out]
                  }
                }
              }
              frame #2 {
                n163 = case shown="True" w282 {
                  tunnel: w281 -> [w286 w296]
                  tunnel: w283 -> [w288 w295]
                  tunnel: w280 -> [w287 w294]
                  tunnel: w279 -> [w289 w299]
                  tunnel: [w286 w293] -> w278
                  tunnel: [w288 w302] -> w277
                  tunnel: [w287 w301] -> w276
                  tunnel: ["Stop" "Connect Weather Station" ("t")] -> w275
                  tunnel: [w289 w299] -> w274
                  tunnel: w273 -> [_ w292]
                  frame False {
                    n164 = call "Status_Error_Message.vi"("Message number"=222) -> ("Status/Error string"=w284:string)
                    n165 = local write "Status/Error messages"(w284) -> ()
                  }
                  frame True {
                    n166 = Unbundle By Name(w299) -> ("Path User Settings file"=w298:path)
                    n167 = case shown="True" w292 {
                      frame False {
                        # "'HELP' button not pressed"
                      }
                      frame True {
                        n168 = stacked-sequence {
                          seq-local: [_ w324 _] -> [_ _ w330]
                          frame #0 {
                            # "'Help' button pressed!"
                            n169 = call "Status_Error_Message.vi"("Message number"=121) -> ("Status/Error string"=w322:string)
                            n170 = local write "Status/Error messages"(w322) -> ()
                          }
                          frame #1 {
                            n171 = global read "Help_URL.vi" "Help URL"() -> (w323:string)
                            n172 = call-poly <vilib>:"Open URL in Default Browser.vi"("URL"=w323) -> ("error out"=w325:errorcluster)  [unwired: 5 in, 1 out]
                            n173 = case shown="No Error" w325 {
                              selector: w325 -> [w326 w327]
                              tunnel: [w326 w327] -> w324
                              frame No Error {
                              }
                              frame Error {
                                # "Cannot reach\nthe internet"
                                n174 = One Button Dialog(message="Error: Cannot start browser/access internet\nor HiSPARC document server off-line! ", button name ("OK")="CONTINUE") -> ()  [unwired: 1 out]
                              }
                            }
                          }
                          frame #2 {
                            n175 = case shown="No Error" w330 {
                              frame No Error {
                                n176 = One Button Dialog(message="When you press 'CONTINUE',\nthe manual remains in your browser!", button name ("OK")="CONTINUE") -> ()  [unwired: 1 out]
                              }
                              frame Error {
                                n177 = call "Status_Error_Message.vi"("Message number"=221) -> ("Status/Error string"=w333:string)
                                n178 = local write "Status/Error messages"(w333) -> ()
                              }
                            }
                          }
                        }
                      }
                    }
                    n179 = stacked-sequence {
                      seq-local: [w304 _ _] -> [_ w314 _]
                      seq-local: [_ w312 _] -> [_ _ w317]
                      tunnel: [_ w311 _] -> w302
                      tunnel: [_ _ w320] -> w301
                      tunnel: w298 -> [w305 _ _]
                      tunnel: w296 -> [w307 _ _]
                      tunnel: w295 -> [_ w311 _]
                      tunnel: w294 -> [_ _ w320]
                      tunnel: [w307 _ _] -> w293
                      frame #0 {
                        n180 = call <vilib>:"Open Config Data.vi"("create file if necessary (T)"=FALSE, "configuration file path"=w305) -> ("refnum"=w306:T4)  [unwired: 7 in, 2 out]
                        n181 = call-poly <vilib>:"Write Key.vi"("section"="Weather" ("key"), "value"=w307, "key"="COM_port", "refnum"=w306) -> ("refnum out"=w304:T4)  [unwired: 5 in, 2 out]
                      }
                      frame #1 {
                        n182 = call-poly <vilib>:"Write Key.vi"("section"="Weather" ("key"), "value"=w311, "key"="Baud_rate", "refnum"=w314) -> ("refnum out"=w312:T4)  [unwired: 5 in, 2 out]
                      }
                      frame #2 {
                        n183 = call-poly <vilib>:"Write Key.vi"("section"="Weather" ("key"), "value"=w320, "key"="Station_ID", "refnum"=w317) -> ("error out"=w315:errorcluster, "refnum out"=w316:T4)  [unwired: 5 in, 1 out]
                        n184 = call <vilib>:"Close Config Data.vi"("error in (no error)"=w315, "refnum"=w316) -> ()  [unwired: 8 in, 2 out]
                      }
                    }
                    n185 = call "Status_Error_Message.vi"("Message number"=122) -> ("Status/Error string"=w297:string)
                    n186 = local write "Status/Error messages"(w297) -> ()
                  }
                }
                n187 = local write "COM port"(w278) -> ()
                n188 = local write "Baud rate"(w277) -> ()
                n189 = local write "Station ID"(w276) -> ()
              }
            }
          }
          frame True {
            n190 = case shown="False" w338 {
              selector: w338 -> [w342 w361]
              tunnel: [w343 w362] -> w339
              tunnel: w337 -> [_ _]
              tunnel: [w342 w361] -> w336
              frame False {
                # "Run-time error occurred:\n- Use the already defined USB/COM port\n- Wait N X 10 seconds (Nmax = 10) to accommodate\n   Windows and/or pc hick-ups\n- Try to establish the connection again"
                n191 = local read "Stop program?"() -> (w341:bool)
                n192 = case shown="False" w341 {
                  tunnel: [w350 "Stop" ("t")] -> w343
                  frame False {
                    n193 = global read "Re_Connection_Counter.vi" "Re-connection counter"() -> (w349:u32)
                    n194 = call "Status_Error_Message.vi"("Message number"=217) -> ("Status/Error string"=w344:string)
                    n195 = local write "Status/Error messages"(w344) -> ()
                    n196 = Multiply(x=w349, y=u32 10000) -> (x*y=w354:u32)
                    n197 = Add(x=w354, y=u32 10000 ("milliseconds to wait")) -> (x+y=w352:u32)
                    n198 = flat-sequence {
                      tunnel: w352 -> [w356]
                      frame #0 {
                        n199 = global read "Re_Connection_Counter.vi" "Re-connection counter"() -> (w357:u32)
                        n200 = Increment(x=w357) -> (x+1=w358:u32)
                        n201 = global write "Re_Connection_Counter.vi" "Re-connection counter"(w358) -> ()
                        n202 = Wait (ms)(milliseconds to wait=w356) -> ()  [unwired: 1 out]
                      }
                    }
                    n203 = Greater Or Equal?(x=w349, y=u32 9) -> (x >= y?=w347:bool)
                    n204 = Select(t="Initialise", s=w347, f="Connect Weather Station" ("t")) -> (s? t:f=w350:string)
                  }
                  frame True {
                  }
                }
              }
              frame True {
                n205 = local read "Stop program?"() -> (w360:bool)
                n206 = case shown="True" w360 {
                  tunnel: ["Get/Set Parameters" ("t") "Stop" ("t")] -> w362
                  frame False {
                    # "Port is open; get/set parameters:\n- Reset run-time error"
                    n207 = global write "Re_Connection_Counter.vi" "Re-connection counter"(u32 0 ("Re-connection counter")) -> ()
                    n208 = local write "Run-time error"(FALSE ("Run-time error")) -> ()
                    n209 = property on="Tab Control" class="TabCtl (strict)"("Visible"=TRUE) -> ()  [unwired: 2 in, 2 out]
                    n210 = call "Status_Error_Message.vi"("Message number"=117) -> ("Status/Error string"=w363:string)
                    n211 = local write "Status/Error messages"(w363) -> ()
                  }
                  frame True {
                  }
                }
              }
            }
            n212 = global read "Status_Error_Messages.vi" "Status/Error messages"() -> (w335:string)
            n213 = local write "Status/Error messages"(w335) -> ()
          }
        }
        "Weather station connected?" <- w218
        n214 = local write "Temperature"(w213) -> ()
        n215 = local write "Humidity"(w213) -> ()
        n216 = local write "Barometer"(w213) -> ()
        n217 = local write "Temperature"(w213) -> ()
        n218 = local write "Humidity"(w213) -> ()
        n219 = local write "Wind direction"(w213) -> ()
        n220 = local write "Wind speed"(w213) -> ()
        n221 = local write "Solar radiation"(w213) -> ()
        n222 = local write "UV index"(w213) -> ()
        n223 = local write "Rain"(w213) -> ()
        n224 = local write "Evapotranspiration"(w213) -> ()
        n225 = local write "Heat index"(w213) -> ()
        n226 = local write "Dew point"(w213) -> ()
        n227 = local write "Wind chill"(w213) -> ()
      }
      frame "Get/Set Parameters" {
        # "Initialisation of the DLL is required since\nit will modify the DLL according to station\ntype and firmware version"
        # "Weather station is connected:\n\n- Set sensor units\n- Synchronise console clock and pc\n- Set calibration values"
        # "Weather station is connected:\n\n- Initialise dll\n- Get weather station model\n- Obtain DLL version\n- Obtain Firmware version\n- Firmware creation date"
        n228 = dll-call lib="C:/Users/SuperUser/Desktop/HiSPARC Weather Station/Develop/VantagePro.dll" fn="_InitStation_V@0" label="InitStation"() -> (error out=w374:errorcluster)  [unwired: 3 in, 2 out]
        n229 = case shown="No Error" w374 {
          tunnel: [w424 "Stop" ("y")] -> w370
          tunnel: [w423 FALSE] -> w375
          frame No Error {
            n230 = call "Weather_Station_Model.vi"() -> ("Supported?"=w421:bool, "Weather station model"=→"Weather station model":string)  [unwired: 1 in]
            n231 = case shown="True" w421 {
              selector: w421 -> [w426 _]
              tunnel: ["Stop" ("y") w431] -> w424
              tunnel: [w426 w430] -> w423
              frame False {
                # "This model weather station is not supported!."
                n232 = call "Status_Error_Message.vi"("Message number"=332) -> ("Status/Error string"=w428:string)
                n233 = local write "Status/Error messages"(w428) -> ()
              }
              frame True {
                n234 = stacked-sequence {
                  seq-local: [w432 _ _ _] -> [_ w435 _ _]
                  seq-local: [_ w434 _ _] -> [_ _ w438 _]
                  seq-local: [_ _ w437 _] -> [_ _ _ w442]
                  tunnel: [_ _ _ w441] -> w429
                  frame #0 {
                    n235 = dll-call lib="C:/Users/SuperUser/Desktop/HiSPARC Weather Station/Develop/VantagePro.dll" fn="_SetVantageTimeoutVal_V@4" label="Set Timeout"("timeOutType"=i16 0) -> (error out=w432:errorcluster)  [unwired: 5 in, 1 out]
                  }
                  frame #1 {
                    n236 = dll-call lib="C:/Users/SuperUser/Desktop/HiSPARC Weather Station/Develop/VantagePro.dll" fn="_GetDllVersion_V@0" label="GetDllVersion"(error in=w435) -> (error out=w434:errorcluster, "return type"=→"DLL Version":sgl)  [unwired: 2 in, 1 out]
                  }
                  frame #2 {
                    n237 = dll-call lib="C:/Users/SuperUser/Desktop/HiSPARC Weather Station/Develop/VantagePro.dll" fn="_GetStationFirmwareVersion_V@4" label="Firmware Version"(error in=w438, "FirmwareVersion"="") -> (error out=w437:errorcluster, "FirmwareVersion"=→"Firmware version":string)  [unwired: 2 in, 2 out]
                  }
                  frame #3 {
                    w445 = "/"
                    n238 = dll-call lib="C:/Users/SuperUser/Desktop/HiSPARC Weather Station/Develop/VantagePro.dll" fn="_GetStationFirmwareDate_V@4" label="Firmware Date"(error in=w442, "FirmwareDate"=cluster{i32, i32, i32, i32, i32} {0, 0, 0, 0, 0} ("Original Console time")) -> (error out=w441:errorcluster, "FirmwareDate"=w450:cluster{i32, i32, i32, i32, i32})  [unwired: 2 in, 2 out]
                    n239 = Unbundle(w450) -> (w449:i32, w444:i32, w443:i32)  [unwired: 2 out]
                    n240 = Number To Decimal String(number=w449) -> (decimal integer string=w448:string)  [unwired: 1 in]
                    n241 = Number To Decimal String(number=w444) -> (decimal integer string=w447:string)  [unwired: 1 in]
                    n242 = Number To Decimal String(number=w443) -> (decimal integer string=w446:string)  [unwired: 1 in]
                    n243 = Concatenate Strings(w448, w445, w447, w445, w446) -> (→"Firmware creation date":string)
                  }
                }
                n244 = case shown="No Error" w429 {
                  tunnel: [w454 "Connect Weather Station"] -> w431
                  tunnel: [w453 FALSE] -> w430
                  frame No Error {
                    w460 = i8 0  # ElevUnit
                    w459 = i8 0  # WindUnit
                    w458 = i8 0  # PressUnit
                    w457 = i8 0  # RainUnit
                    w456 = i8 0  # TempUnit
                    # "Sensor units:\n- Fahrenheit\n- inches\n- inches\n- miles/hr\n- feet"
                    n245 = Bundle("TempUnit"=w456, "RainUnit"=w457, "PressUnit"=w458, "WindUnit"=w459, "ElevUnit"=w460) -> (w461:T5)  [unwired: 1 out]
                    n246 = call "Set_Sensor_Units.vi"("Weather sensor units"=w461) -> ("Succes?"=w455:bool)
                    n247 = case shown="True" w455 {
                      selector: w455 -> [w464 _]
                      tunnel: [w464 w468] -> w453
                      tunnel: ["Connect Weather Station" w469] -> w454
                      frame False {
                        # "Cannot initialise sensor units"
                        n248 = flat-sequence {
                          frame #0 {
                            n249 = call "Status_Error_Message.vi"("Message number"=232) -> ("Status/Error string"=w465:string)
                            n250 = local write "Status/Error messages"(w465) -> ()
                          }
                          frame #1 {
                            # "Close connection"
                            n251 = call "Close_WeatherStation_Connection.vi"() -> ("Status/Error string"=w467:string)
                            n252 = local write "Status/Error messages"(w467) -> ()
                          }
                        }
                        n253 = local write "Run-time error"(TRUE ("Run-time error")) -> ()
                      }
                      frame True {
                        # "0.2 mm"
                        n254 = call "Set_Rain_CupSize.vi"("Rain cup size"=i16 2 ("0.2 mm")) -> ("Succes?"=w470:bool)
                        n255 = case shown="True" w470 {
                          selector: w470 -> [w472 _]
                          tunnel: ["Connect Weather Station" w481] -> w469
                          tunnel: [w472 w480] -> w468
                          frame False {
                            n256 = flat-sequence {
                              frame #0 {
                                n257 = call "Status_Error_Message.vi"("Message number"=233) -> ("Status/Error string"=w476:string)
                                n258 = local write "Status/Error messages"(w476) -> ()
                              }
                              frame #1 {
                                # "Close connection"
                                n259 = call "Close_WeatherStation_Connection.vi"() -> ("Status/Error string"=w477:string)
                                n260 = local write "Status/Error messages"(w477) -> ()
                              }
                            }
                            n261 = local write "Run-time error"(TRUE ("Run-time error")) -> ()
                          }
                          frame True {
                            # "Large"
                            n262 = call "Set_Wind_CupSize.vi"("Wind cup size"=i16 2) -> ("Succes?"=w479:bool)
                            n263 = case shown="True" w479 {
                              selector: w479 -> [w482 _]
                              tunnel: ["Connect Weather Station" w489] -> w481
                              tunnel: [w482 w488] -> w480
                              frame False {
                                n264 = flat-sequence {
                                frame #0 {
                                n265 = call "Status_Error_Message.vi"("Message number"=234) -> ("Status/Error string"=w486:string)
                                n266 = local write "Status/Error messages"(w486) -> ()
                                }
                                frame #1 {
                                # "Close connection"
                                n267 = call "Close_WeatherStation_Connection.vi"() -> ("Status/Error string"=w487:string)
                                n268 = local write "Status/Error messages"(w487) -> ()
                                }
                                }
                                n269 = local write "Run-time error"(TRUE ("Run-time error")) -> ()
                              }
                              frame True {
                                # "Synchronise\nclocks"
                                n270 = call "Synchronise_Console_PC.vi"() -> ("PC_time = Console_time?"=w490:bool)
                                n271 = case shown="True" w490 {
                                selector: w490 -> [w491 w497]
                                tunnel: ["Connect Weather Station" w499] -> w489
                                tunnel: [w491 w497] -> w488
                                frame False {
                                n272 = flat-sequence {
                                frame #0 {
                                n273 = call "Status_Error_Message.vi"("Message number"=235) -> ("Status/Error string"=w494:string)
                                n274 = local write "Status/Error messages"(w494) -> ()
                                }
                                frame #1 {
                                # "Close connection"
                                n275 = call "Close_WeatherStation_Connection.vi"() -> ("Status/Error string"=w496:string)
                                n276 = local write "Status/Error messages"(w496) -> ()
                                }
                                }
                                n277 = local write "Run-time error"(TRUE ("Run-time error")) -> ()
                                }
                                frame True {
                                # "Station GPS\ncoordinates"
                                n278 = global read "Station_Coordinates.vi" "Station latitude"() -> (w502:dbl)
                                n279 = global read "Station_Coordinates.vi" "Station longitude"() -> (w501:dbl)
                                n280 = call "Set_Coordinates.vi"("Longitude"=w501, "Latitude"=w502, "Degrees?"=FALSE, "Path"=path "") -> ("Succes?"=w500:bool)
                                n281 = case shown="True" w500 {
                                tunnel: ["Connect Weather Station" w509] -> w499
                                frame False {
                                n282 = stacked-sequence {
                                frame #0 {
                                n283 = call "Status_Error_Message.vi"("Message number"=236) -> ("Status/Error string"=w506:string)
                                n284 = local write "Status/Error messages"(w506) -> ()
                                }
                                frame #1 {
                                # "Close connection"
                                n285 = call "Close_WeatherStation_Connection.vi"() -> ("Status/Error string"=w508:string)
                                n286 = local write "Status/Error messages"(w508) -> ()
                                }
                                }
                                n287 = local write "Run-time error"(TRUE) -> ()
                                }
                                frame True {
                                n288 = global read "Barometer_Calibration.vi" "Barometer sea level [hPa]"() -> (w513:dbl)
                                n289 = global read "Barometer_Calibration.vi" "Station elevation [m]"() -> (w512:i32)
                                n290 = call "Set_Barometer_Calibration.vi"("Elevation"=w512, "Sea level in"=w513, "Path"=path "") -> ("Calibration values set?"=w510:bool)  [unwired: 1 out]
                                n291 = case shown="True" w510 {
                                tunnel: ["Connect Weather Station" "Read Weather Data"] -> w509
                                frame False {
                                n292 = stacked-sequence {
                                frame #0 {
                                n293 = call "Status_Error_Message.vi"("Message number"=237) -> ("Status/Error string"=w516:string)
                                n294 = local write "Status/Error messages"(w516) -> ()
                                }
                                frame #1 {
                                n295 = call "Close_WeatherStation_Connection.vi"() -> ("Status/Error string"=w518:string)
                                n296 = local write "Status/Error messages"(w518) -> ()
                                }
                                }
                                n297 = local write "Run-time error"(TRUE) -> ()
                                }
                                frame True {
                                }
                                }
                                }
                                }
                                }
                                }
                              }
                            }
                          }
                        }
                      }
                    }
                  }
                  frame Error {
                    # "Failed to get DLL/Firmware info and/orfirmware date"
                    n298 = flat-sequence {
                      frame #0 {
                        n299 = call "Status_Error_Message.vi"("Message number"=231) -> ("Status/Error string"=w523:string)
                        n300 = local write "Status/Error messages"(w523) -> ()
                      }
                      frame #1 {
                        # "Close connection"
                        n301 = call "Close_WeatherStation_Connection.vi"() -> ("Status/Error string"=w525:string)
                        n302 = local write "Status/Error messages"(w525) -> ()
                      }
                    }
                    n303 = local write "Run-time error"(TRUE ("Run-time error")) -> ()
                  }
                }
              }
            }
          }
          frame Error {
            # "Error initialising supporting DLL."
            n304 = call "Status_Error_Message.vi"("Message number"=331) -> ("Status/Error string"=w528:string)
            n305 = local write "Status/Error messages"(w528) -> ()
          }
        }
        "PC time =\nConsole time?" <- w375
        n306 = Equal?(x=w370, y="Read Weather Data") -> (x = y?=w372:bool)
        n307 = case shown="True" w372 {
          tunnel: [w379 w395] -> w371
          tunnel: w370 -> [w378 w395]
          frame False {
            w377 = FALSE ("Weather station connected?")
            n308 = Equal?(x=w378, y="Stop") -> (x = y?=w380:bool)
            n309 = case shown="False" w380 {
              tunnel: [w383 w394] -> w379
              tunnel: w378 -> [w382 w394]
              frame False {
                # "Either there are problems with\nthe initialisation of parameters\nof the station or DAQ is quit\n(fatal error?)..."
                n310 = global read "Re_Initialisation_Counter.vi" "Re-initialisation counter"() -> (w387:u32)
                n311 = Increment(x=w387) -> (x+1=w385:u32)
                n312 = Greater Or Equal?(x=w385, y=u32 3) -> (x >= y?=w384:bool)
                n313 = global write "Re_Initialisation_Counter.vi" "Re-initialisation counter"(w385) -> ()
                n314 = case shown="True" w384 {
                  tunnel: [w390 "Stop"] -> w383
                  tunnel: w382 -> [w390 _]
                  frame False {
                    n315 = call "Status_Error_Message.vi"("Message number"=230) -> ("Status/Error string"=w388:string)
                    n316 = local write "Status/Error messages"(w388) -> ()
                  }
                  frame True {
                    n317 = call "Status_Error_Message.vi"("Message number"=330) -> ("Status/Error string"=w392:string)
                    n318 = local write "Status/Error messages"(w392) -> ()
                  }
                }
              }
              frame True {
                # "Quit"
              }
            }
            n319 = local write "Weather station connected?"(w377) -> ()
            n320 = local write "PC time =\nConsole time?"(w377) -> ()
          }
          frame True {
            n321 = stacked-sequence {
              frame #0 {
                # "Clear console data logger memory"
                n322 = dll-call lib="C:/Users/SuperUser/Desktop/HiSPARC Weather Station/Develop/VantagePro.dll" fn="_ClearStoredData_V@0" label="Clear Stored Data"() -> (error out=w396:errorcluster)  [unwired: 4 in, 1 out]
                n323 = case shown="No Error" w396 {
                  frame No Error {
                    n324 = call "Status_Error_Message.vi"("Message number"=118) -> ("Status/Error string"=w397:string)
                    n325 = local write "Status/Error messages"(w397) -> ()
                  }
                  frame Error {
                    n326 = call "Status_Error_Message.vi"("Message number"=218) -> ("Status/Error string"=w399:string)
                    n327 = local write "Status/Error messages"(w399) -> ()
                  }
                }
              }
              frame #1 {
                # "Weather station console initialised"
                n328 = call "Status_Error_Message.vi"("Message number"=131) -> ("Status/Error string"=w401:string)
                n329 = local write "Status/Error messages"(w401) -> ()
              }
              frame #2 {
                w403 = TRUE ("Visible")
                n330 = local read "DAQ mode?"() -> (w408:bool)
                n331 = property on="Tab Control" class="TabCtl (strict)"() -> ("Pages"=w407:refnum<vi>[])  [unwired: 2 in, 2 out]
                n332 = property on="DAQ software version" class="Str"("Visible"=w403) -> ()  [unwired: 2 in, 2 out]
                n333 = case shown="True" w408 {
                  tunnel: w407 -> [w412 w415]
                  tunnel: [bool[] [TRUE, TRUE, TRUE, TRUE, TRUE] bool[] [TRUE, TRUE, TRUE, TRUE, FALSE]] -> w406
                  tunnel: [w412 w415] -> w405
                  tunnel: [TRUE FALSE] -> w404
                  frame False {
                  }
                  frame True {
                  }
                }
                n334 = property on="DAQ mode?" class="Bool (strict)"("Visible"=w403) -> ()  [unwired: 2 in, 2 out]
                n335 = for {
                  tunnel: [w409] -> _ mode=indexing
                  tunnel: w406 -> [w410] mode=indexing
                  tunnel: w405 -> [w409] mode=indexing
                  n336 = property class="Page"(reference=w409, "PageVis"=w410) -> ()  [unwired: 1 in, 2 out]
                }
                n337 = property on="Help?" class="Bool (strict)"("Visible"=w404) -> ()  [unwired: 2 in, 2 out]
                n338 = property on="Stop program?" class="Bool (strict)"("Visible"=w404) -> ()  [unwired: 2 in, 2 out]
                n339 = property on="Tab Control" class="TabCtl (strict)"("Visible"=w403) -> ()  [unwired: 2 in, 2 out]
              }
              frame #3 {
                # "Display USB or Serial connection"
                n340 = global read "USB_WeatherLink_Serialnumber.vi" "WeatherLink USB serial number"() -> (w419:u32)
                "USB Weather Link" <- w419
                n341 = Not Equal To 0?(x=w419) -> (x != 0?=w417:bool)
                n342 = Not(x=w417) -> (.not. x?=w418:bool)
                n343 = property on="USB Weather Link" class="DigNum (strict)"("Visible"=w417) -> ()  [unwired: 2 in, 2 out]
                n344 = property on="COM port" class="DigNum (strict)"("Visible"=w418) -> ()  [unwired: 2 in, 2 out]
                n345 = property on="Baud rate" class="DigNum (strict)"("Visible"=w418) -> ()  [unwired: 2 in, 2 out]
              }
              frame #4 {
                n346 = Get Date/Time In Seconds() -> (seconds since 1Jan1904=→"Start-time data taking":timestamp)
              }
            }
          }
        }
      }
      frame "Read Weather Data" {
        # "There are 4 main execution loops here:\n\n- loop waiting for front panel input (top)\n- average 60 s, update graphs (middle, 1 and 48 hrs data)\n- submit 5 seconds data to the data buffer ( left)\n- loop for data taking (bottom, 1 event/ 5 seconds)"
        n347 = Get Date/Time In Seconds() -> (seconds since 1Jan1904=w533:timestamp)
        n348 = while {
          tunnel: [w1008] -> w534
          shift-right: [w1011] -> w539
          shift-left: w530 -> [w1010]
          stop <- w1005 stop-if-true
          # "Front\npanel:\n(Stop)\nDAQ?"
          n349 = case shown="False" "DAQ mode?" {
            tunnel: w1010 -> [w1016 w1326]
            tunnel: [w1015 "Read Weather Data" ("y")] -> w1008
            tunnel: [w1014 w1326] -> w1011
            frame False {
              # "Front\npanel:\nStop?"
              n350 = case shown="False" "Stop program?" {
                tunnel: w1016 -> [w1020 w1322]
                tunnel: [w1018 "Stop" ("y")] -> w1015
                tunnel: [w1019 w1322] -> w1014
                frame False {
                  # "Front\npanel:\nSave\nSettings?"
                  n351 = case shown="False" "Save settings?" {
                    tunnel: w1020 -> [w1022 w1257]
                    tunnel: [w1021 w1257] -> w1019
                    tunnel: [w1024 "Read Weather Data" ("y")] -> w1018
                    frame False {
                      # "Front\npanel:\nSave\nCalibr?"
                      n352 = case shown="False" "Save calibration?" {
                        tunnel: [w1026 w1079] -> w1024
                        tunnel: w1022 -> [w1025 w1078]
                        tunnel: [w1025 w1078] -> w1021
                        frame False {
                          # "Front\npanel:\nReset?"
                          n353 = case shown="True" "Reset settings?" {
                            tunnel: [w1029 w1054] -> w1026
                            tunnel: w1025 -> [_ w1057]
                            frame False {
                              # "Front\npanel:\nHelp?"
                              n354 = case shown="False" "Help?" {
                                tunnel: ["Read Weather Data" ("y") "Read Weather Data" ("y")] -> w1029
                                frame False {
                                n355 = global read "DAQ_Mode.vi" "DAQ mode?"() -> (w1031:bool)
                                n356 = case shown="False" w1031 {
                                frame False {
                                # "Do nothing as the DAQ is NOT\ntransferring data to the buffer"
                                }
                                frame True {
                                w1033 = TRUE ("Visible")
                                # "Stop transfer to buffer; show buttons"
                                n357 = property on="Tab Control" class="TabCtl (strict)"() -> ("Pages"=w1035:refnum<vi>[])  [unwired: 2 in, 2 out]
                                n358 = for {
                                tunnel: w1035 -> [w1039] mode=indexing
                                tunnel: bool[] [TRUE, TRUE, TRUE, TRUE, TRUE] -> [w1038] mode=indexing
                                n359 = property class="Page"(reference=w1039, "PageVis"=w1038) -> ()  [unwired: 1 in, 2 out]
                                }
                                n360 = property on="Stop program?" class="Bool (strict)"("Visible"=w1033) -> ()  [unwired: 2 in, 2 out]
                                n361 = property on="Help?" class="Bool (strict)"("Visible"=w1033) -> ()  [unwired: 2 in, 2 out]
                                n362 = call "Status_Error_Message.vi"("Message number"=130) -> ("Status/Error string"=w1034:string)
                                n363 = global write "DAQ_Mode.vi" "DAQ mode?"(FALSE ("DAQ mode?")) -> ()
                                n364 = local write "Status/Error messages"(w1034) -> ()
                                }
                                }
                                }
                                frame True {
                                # "Open web page with instructions"
                                n365 = local write "Help?"(FALSE ("Save calibration?")) -> ()
                                n366 = stacked-sequence {
                                frame #0 {
                                w1043 = FALSE ("Start/Stop message?")
                                n367 = call "Status_Error_Message.vi"("Message number"=129) -> ("Status/Error string"=w1044:string)
                                n368 = property on="Tab Control" class="TabCtl (strict)"("Visible"=w1043) -> ()  [unwired: 2 in, 2 out]
                                n369 = property on="Stop program?" class="Bool (strict)"("Visible"=w1043) -> ()  [unwired: 2 in, 2 out]
                                n370 = local write "Status/Error messages"(w1044) -> ()
                                n371 = property on="DAQ mode?" class="Bool (strict)"("Visible"=w1043) -> ()  [unwired: 2 in, 2 out]
                                n372 = property on="DAQ software version" class="Str"("Visible"=w1043) -> ()  [unwired: 2 in, 2 out]
                                n373 = property on="Help?" class="Bool (strict)"("Visible"=w1043) -> ()  [unwired: 2 in, 2 out]
                                }
                                frame #1 {
                                n374 = global read "Help_URL.vi" "Help URL"() -> (w1045:string)
                                n375 = call-poly <vilib>:"Open URL in Default Browser.vi"("URL"=w1045) -> ("error out"=w1046:errorcluster)  [unwired: 5 in, 1 out]
                                n376 = case shown="No Error" w1046 {
                                frame No Error {
                                n377 = One Button Dialog(message="When you press 'CONTINUE',\nthe manual remains in your browser!", button name ("OK")="CONTINUE") -> ()  [unwired: 1 out]
                                }
                                frame Error {
                                # "Cannot reach\nthe internet"
                                n378 = One Button Dialog(message="Error: Cannot start browser/access internet\nor HiSPARC document server off-line! ", button name ("OK")="CONTINUE") -> ()  [unwired: 1 out]
                                }
                                }
                                }
                                frame #2 {
                                w1051 = TRUE ("Visible")
                                n379 = property on="Stop program?" class="Bool (strict)"("Visible"=w1051) -> ()  [unwired: 2 in, 2 out]
                                n380 = property on="Tab Control" class="TabCtl (strict)"("Visible"=w1051) -> ()  [unwired: 2 in, 2 out]
                                n381 = property on="Help?" class="Bool (strict)"("Visible"=w1051) -> ()  [unwired: 2 in, 2 out]
                                n382 = property on="DAQ software version" class="Str"("Visible"=w1051) -> ()  [unwired: 2 in, 2 out]
                                n383 = property on="DAQ mode?" class="Bool (strict)"("Visible"=w1051) -> ()  [unwired: 2 in, 2 out]
                                }
                                }
                                }
                              }
                            }
                            frame True {
                              n384 = flat-sequence {
                                tunnel: w1057 -> [w1063]
                                tunnel: [w1063] -> w1056
                                frame #0 {
                                w1062 = FALSE ("Visible")
                                n385 = property on="Tab Control" class="TabCtl (strict)"("Visible"=w1062) -> ()  [unwired: 2 in, 2 out]
                                n386 = property on="Stop program?" class="Bool (strict)"("Visible"=w1062) -> ()  [unwired: 2 in, 2 out]
                                n387 = property on="DAQ mode?" class="Bool (strict)"("Visible"=w1062) -> ()  [unwired: 2 in, 2 out]
                                n388 = property on="Help?" class="Bool (strict)"("Visible"=w1062) -> ()  [unwired: 2 in, 2 out]
                                n389 = property on="DAQ software version" class="Str"("Visible"=w1062) -> ()  [unwired: 2 in, 2 out]
                                }
                              }
                              n390 = Two Button Dialog(message="Do you realy wish to reset to default settings?\nUser settings will be lost!", 1:"NO" ("F button name (\"Cancel\")"), 2:"YES" ("T button name (\"OK\")")) -> (T button?=w1058:bool)
                              n391 = case shown="True" w1058 {
                                tunnel: ["Read Weather Data" ("y") "Initialise"] -> w1055
                                tunnel: w1056 -> [_ w1068]
                                frame False {
                                # "Ignore RESET; continue data taking"
                                n392 = call "Status_Error_Message.vi"("Message number"=128) -> ("Status/Error string"=w1066:string)
                                n393 = local write "Reset settings?"(FALSE ("Reset settings?")) -> ()
                                n394 = local write "Status/Error messages"(w1066) -> ()
                                }
                                frame True {
                                # "Reset: Delete user file, Reset cal. values,\nClose port, re-start with default settings"
                                n395 = stacked-sequence {
                                tunnel: w1068 -> [w1070 _ _ _]
                                frame #0 {
                                n396 = Unbundle By Name(w1070) -> ("Path User Settings file"=w1071:path)
                                n397 = local write "Reset settings?"(FALSE ("Reset settings?")) -> ()
                                n398 = Delete(path (use dialog)=w1071) -> ()  [unwired: 4 in, 3 out]
                                }
                                frame #1 {
                                n399 = dll-call lib="C:/Users/SuperUser/Desktop/HiSPARC Weather Station/Develop/VantagePro.dll" fn="_ClearVantageCalNums_V@0" ("Clear Cal Nums")() -> (error out=w1073:errorcluster)  [unwired: 4 in, 1 out]
                                n400 = case shown="No Error" w1073 {
                                frame No Error {
                                n401 = dll-call lib="C:/Users/SuperUser/Desktop/HiSPARC Weather Station/Develop/VantagePro.dll" fn="_InitStation_V@0" label="InitStation"() -> (error out=w1074:errorcluster)  [unwired: 3 in, 2 out]
                                n402 = case shown="No Error" w1074 {
                                frame No Error {
                                }
                                frame Error {
                                }
                                }
                                }
                                frame Error {
                                }
                                }
                                }
                                frame #2 {
                                n403 = call "Status_Error_Message.vi"("Message number"=228) -> ("Status/Error string"=w1076:string)
                                n404 = local write "Status/Error messages"(w1076) -> ()
                                }
                                frame #3 {
                                n405 = call "Close_WeatherStation_Connection.vi"() -> ("Status/Error string"=w1077:string)
                                n406 = local write "Status/Error messages"(w1077) -> ()
                                }
                                }
                                }
                              }
                              n407 = flat-sequence {
                                tunnel: w1055 -> [w1061]
                                tunnel: [w1061] -> w1054
                                frame #0 {
                                w1060 = TRUE ("Visible")
                                n408 = property on="Tab Control" class="TabCtl (strict)"("Visible"=w1060) -> ()  [unwired: 2 in, 2 out]
                                n409 = property on="Stop program?" class="Bool (strict)"("Visible"=w1060) -> ()  [unwired: 2 in, 2 out]
                                n410 = property on="DAQ mode?" class="Bool (strict)"("Visible"=w1060) -> ()  [unwired: 2 in, 2 out]
                                n411 = property on="Help?" class="Bool (strict)"("Visible"=w1060) -> ()  [unwired: 2 in, 2 out]
                                n412 = property on="DAQ software version" class="Str"("Visible"=w1060) -> ()  [unwired: 2 in, 2 out]
                                }
                              }
                            }
                          }
                        }
                        frame True {
                          n413 = stacked-sequence {
                            seq-local: [w1080 _ _ _ _ _] -> [_ w1100 w1121 w1200 w1232 _]
                            seq-local: [_ _ _ w1197 _ _] -> [_ _ _ _ _ w1249]
                            seq-local: [_ w1094 _ _ _ _] -> [_ _ _ _ _ w1250]
                            seq-local: [_ _ w1120 _ _ _] -> [_ _ _ _ _ w1251]
                            seq-local: [_ _ _ _ w1224 _] -> [_ _ _ _ _ w1247]
                            tunnel: [_ _ _ _ _ w1252] -> w1079
                            tunnel: w1078 -> [_ w1098 w1160 w1204 w1226 _]
                            frame #0 {
                              n414 = flat-sequence {
                                tunnel: [w1085] -> w1080
                                frame #0 {
                                w1082 = FALSE ("Visible")
                                # "'SAVE CALIBRATION'"
                                n415 = property on="Tab Control" class="TabCtl (strict)"("Visible"=w1082) -> ()  [unwired: 2 in, 2 out]
                                n416 = call "Status_Error_Message.vi"("Message number"=126) -> ("Status/Error string"=w1083:string)
                                n417 = property on="Stop program?" class="Bool (strict)"("Visible"=w1082) -> ()  [unwired: 2 in, 2 out]
                                n418 = local write "Status/Error messages"(w1083) -> ()
                                n419 = local write "Save calibration?"(FALSE ("Save calibration?")) -> ()
                                n420 = property on="DAQ mode?" class="Bool (strict)"("Visible"=w1082) -> ()  [unwired: 2 in, 2 out]
                                n421 = property on="Help?" class="Bool (strict)"("Visible"=w1082) -> ()  [unwired: 2 in, 2 out]
                                n422 = property on="DAQ software version" class="Str"("Visible"=w1082) -> ()  [unwired: 2 in, 2 out]
                                }
                                frame #1 {
                                n423 = Two Button Dialog(message="Use this option with care (read instructions!):\nDo you really wish to change the calibration settings?", 1:"NO" ("F button name (\"Cancel\")"), 2:"YES" ("T button name (\"OK\")")) -> (T button?=w1086:bool)
                                n424 = case shown="False" w1086 {
                                selector: w1086 -> [w1092 w1093]
                                tunnel: [w1092 w1093] -> w1085
                                frame False {
                                # "Calibration ignored"
                                n425 = call "Status_Error_Message.vi"("Message number"=127) -> ("Status/Error string"=w1091:string)
                                n426 = local write "Status/Error messages"(w1091) -> ()
                                }
                                frame True {
                                }
                                }
                                }
                              }
                            }
                            frame #1 {
                              n427 = Unbundle By Name(w1098) -> ("Path User Settings file"=w1097:path)
                              n428 = global read "Station_Coordinates.vi" "Station latitude"() -> (w1103:dbl)
                              n429 = global read "Station_Coordinates.vi" "Station longitude"() -> (w1102:dbl)
                              n430 = Not Equal?(x="Latitude [º]", y=w1103) -> (x != y?=w1104:bool)
                              n431 = Not Equal?(x=w1102, y="Longitude [º]") -> (x != y?=w1105:bool)
                              n432 = Or(x=w1104, y=w1105) -> (x .or. y?=w1101:bool)
                              n433 = And(x=w1100, y=w1101) -> (x .and. y?=w1099:bool)
                              n434 = case shown="True" w1099 {
                                tunnel: w1097 -> [_ w1112]
                                tunnel: "Latitude [º]" -> [_ w1109]
                                tunnel: "Longitude [º]" -> [_ w1110]
                                tunnel: [TRUE ("Succes?") w1111] -> w1094
                                frame False {
                                # "No changes"
                                n435 = call "Status_Error_Message.vi"("Message number"=136) -> ("Status/Error string"=w1106:string)
                                n436 = local write "Status/Error messages"(w1106) -> ()
                                }
                                frame True {
                                n437 = call "Set_Coordinates.vi"("Longitude"=w1110, "Latitude"=w1109, "Degrees?"=FALSE, "Path"=w1112) -> ("Succes?"=w1111:bool)
                                n438 = case shown="True" w1111 {
                                tunnel: w1110 -> [_ w1117]
                                tunnel: w1109 -> [_ w1116]
                                frame False {
                                # "Failed to modify latitude and/or longitude"
                                n439 = call "Status_Error_Message.vi"("Message number"=336) -> ("Status/Error string"=w1114:string)
                                n440 = local write "Status/Error messages"(w1114) -> ()
                                }
                                frame True {
                                # "Latitude and/or longitude modified"
                                n441 = global write "Station_Coordinates.vi" "Station latitude"(w1116) -> ()
                                n442 = global write "Station_Coordinates.vi" "Station longitude"(w1117) -> ()
                                n443 = call "Status_Error_Message.vi"("Message number"=236) -> ("Status/Error string"=w1118:string)
                                n444 = local write "Status/Error messages"(w1118) -> ()
                                }
                                }
                                }
                              }
                            }
                            frame #2 {
                              w1155 = 7.0 ("x")
                              n445 = local read "Temp in [°C]"() -> (w1149:dbl)
                              n446 = local read "Temp out [°C]"() -> (w1143:dbl)
                              n447 = local read "Hum in [%]"() -> (w1150:dbl)
                              n448 = local read "Hum out [%]"() -> (w1151:dbl)
                              n449 = Add(x=w1155, y=w1149) -> (x+y=w1158:dbl)
                              n450 = Subtract(x=w1149, y=w1155) -> (x-y=w1157:dbl)
                              n451 = Add(x=w1155, y=w1143) -> (x+y=w1154:dbl)
                              n452 = Subtract(x=w1143, y=w1155) -> (x-y=w1156:dbl)
                              n453 = Unbundle By Name(w1160) -> ("Path User Settings file"=w1159:path)
                              n454 = Not A Number/Path/Refnum?(number/path/refnum=w1150) -> (NaN/Path/Refnum?=w1140:bool)
                              n455 = Not A Number/Path/Refnum?(number/path/refnum=w1151) -> (NaN/Path/Refnum?=w1138:bool)
                              n456 = Not A Number/Path/Refnum?(number/path/refnum="Cal. outside hum. [%]") -> (NaN/Path/Refnum?=w1135:bool)
                              n457 = Not(x=w1140) -> (.not. x?=w1139:bool)
                              n458 = Not(x=w1138) -> (.not. x?=w1136:bool)
                              n459 = In Range and Coerce(upper limit=w1158, x="Cal. inside temp. [°C]", lower limit=w1157) -> (coerced(x)=w1152:dbl)  [unwired: 1 out]
                              n460 = In Range and Coerce(upper limit=w1154, x="Cal. outside temp. [°C]", lower limit=w1156) -> (coerced(x)=w1144:dbl)  [unwired: 1 out]
                              n461 = Not(x=w1135) -> (.not. x?=w1134:bool)
                              n462 = Not A Number/Path/Refnum?(number/path/refnum=w1143) -> (NaN/Path/Refnum?=w1145:bool)
                              n463 = Not A Number/Path/Refnum?(number/path/refnum="Cal. inside temp. [°C]") -> (NaN/Path/Refnum?=w1130:bool)
                              n464 = Not A Number/Path/Refnum?(number/path/refnum="Cal. inside hum. [%]") -> (NaN/Path/Refnum?=w1127:bool)
                              n465 = And(x=w1136, y=w1134) -> (x .and. y?=w1137:bool)
                              n466 = Not(x=w1145) -> (.not. x?=w1142:bool)
                              n467 = Not(x=w1127) -> (.not. x?=w1133:bool)
                              n468 = Not(x=w1130) -> (.not. x?=w1128:bool)
                              n469 = Not A Number/Path/Refnum?(number/path/refnum="Cal. outside temp. [°C]") -> (NaN/Path/Refnum?=w1132:bool)
                              n470 = Not A Number/Path/Refnum?(number/path/refnum=w1149) -> (NaN/Path/Refnum?=w1148:bool)
                              n471 = And(x=w1139, y=w1133) -> (x .and. y?=w1141:bool)
                              n472 = Not(x=w1132) -> (.not. x?=w1131:bool)
                              n473 = Not(x=w1148) -> (.not. x?=w1129:bool)
                              n474 = And(x=w1129, y=w1128) -> (x .and. y?=w1147:bool)
                              n475 = And(x=w1131, y=w1142) -> (x .and. y?=w1146:bool)
                              n476 = Compound Arithmetic op=OR(w1147, w1146, w1141, w1137) -> (w1122:bool)
                              n477 = And(x=w1121, y=w1122) -> (x .and. y?=w1153:bool)
                              n478 = case shown="True" w1153 {
                                tunnel: w1159 -> [_ w1165]
                                tunnel: [TRUE ("Succes?") w1166] -> w1120
                                tunnel: w1152 -> [_ w1169]
                                tunnel: w1144 -> [_ w1170]
                                tunnel: "Cal. inside hum. [%]" -> [_ w1168]
                                tunnel: "Cal. outside hum. [%]" -> [_ w1167]
                                frame False {
                                # "No changes"
                                n479 = call "Status_Error_Message.vi"("Message number"=137) -> ("Status/Error string"=w1161:string)
                                n480 = local write "Status/Error messages"(w1161) -> ()
                                }
                                frame True {
                                n481 = dll-call lib="C:/Users/SuperUser/Desktop/HiSPARC Weather Station/Develop/VantagePro.dll" fn="_ClearVantageCalNums_V@0" ("Clear Cal Nums")() -> (error out=w1164:errorcluster)  [unwired: 4 in, 1 out]
                                n482 = case shown="No Error" w1164 {
                                tunnel: w1170 -> [w1179 _]
                                tunnel: w1169 -> [w1180 _]
                                tunnel: w1168 -> [w1178 _]
                                tunnel: w1167 -> [w1177 _]
                                tunnel: [w1171 FALSE ("Calibration values set?")] -> w1166
                                tunnel: w1165 -> [w1176 _]
                                frame No Error {
                                n483 = call "Set_TempHum_Calibration.vi"("Path"=w1176, "Inside temp"=w1180, "Outside temp"=w1179, "Inside hum."=w1178, "Outside hum"=w1177) -> ("Cor. in temp"=w1175:dbl, "Cor. out temp"=w1174:dbl, "Cor. in hum"=w1173:dbl, "Cor. out hum"=w1172:dbl, "Calibration values set?"=w1171:bool)
                                n484 = case shown="True" w1171 {
                                tunnel: w1175 -> [_ w1186]
                                tunnel: w1174 -> [_ w1185]
                                tunnel: w1173 -> [_ w1184]
                                tunnel: w1172 -> [_ w1183]
                                frame False {
                                n485 = call "Status_Error_Message.vi"("Message number"=337) -> ("Status/Error string"=w1181:string)
                                n486 = local write "Status/Error messages"(w1181) -> ()
                                }
                                frame True {
                                n487 = stacked-sequence {
                                tunnel: w1186 -> [w1190 _]
                                tunnel: w1185 -> [w1189 _]
                                tunnel: w1184 -> [w1188 _]
                                tunnel: w1183 -> [w1187 _]
                                frame #0 {
                                "Cur out hum" <- w1187
                                "Cur in temp" <- w1190
                                "Cur in hum" <- w1188
                                "Cur out temp" <- w1189
                                }
                                frame #1 {
                                w1191 = nan ("Data_input")
                                n488 = call "Status_Error_Message.vi"("Message number"=327) -> ("Status/Error string"=w1192:string)
                                n489 = local write "Cal. inside temp. [°C]"(w1191) -> ()
                                n490 = local write "Cal. outside temp. [°C]"(w1191) -> ()
                                n491 = local write "Cal. inside hum. [%]"(w1191) -> ()
                                n492 = local write "Cal. outside hum. [%]"(w1191) -> ()
                                n493 = local write "Status/Error messages"(w1192) -> ()
                                }
                                }
                                }
                                }
                                }
                                frame Error {
                                n494 = call "Status_Error_Message.vi"("Message number"=338) -> ("Status/Error string"=w1194:string)
                                n495 = local write "Status/Error messages"(w1194) -> ()
                                }
                                }
                                }
                              }
                            }
                            frame #3 {
                              n496 = Unbundle By Name(w1204) -> ("Path User Settings file"=w1203:path)
                              n497 = global read "TempHumWindDir_Calibration.vi" "Wind dir."() -> (w1202:i32)
                              n498 = Not Equal?(x=w1202, y="Offset wind dir. [º]") -> (x != y?=w1199:bool)
                              n499 = And(x=w1200, y=w1199) -> (x .and. y?=w1198:bool)
                              n500 = case shown="True" w1198 {
                                tunnel: w1203 -> [_ w1210]
                                tunnel: [TRUE ("Succes?") w1209] -> w1197
                                tunnel: "Offset wind dir. [º]" -> [_ w1208]
                                frame False {
                                # "No changes"
                                n501 = call "Status_Error_Message.vi"("Message number"=139) -> ("Status/Error string"=w1205:string)
                                n502 = local write "Status/Error messages"(w1205) -> ()
                                }
                                frame True {
                                n503 = call "Set_WindDir_Calibration.vi"("Wind dir off"=w1208, "Path"=w1210) -> ("Calibration value set?"=w1209:bool)
                                n504 = case shown="True" w1209 {
                                tunnel: w1208 -> [_ w1213]
                                frame False {
                                n505 = call "Status_Error_Message.vi"("Message number"=339) -> ("Status/Error string"=w1211:string)
                                n506 = local write "Status/Error messages"(w1211) -> ()
                                }
                                frame True {
                                n507 = stacked-sequence {
                                tunnel: w1213 -> [w1214 _ _]
                                frame #0 {
                                n508 = global write "TempHumWindDir_Calibration.vi" "Wind dir."(w1214) -> ()
                                }
                                frame #1 {
                                n509 = local read "Wind direction"() -> (w1219:bool)
                                n510 = dll-call lib="C:/Users/SuperUser/Desktop/HiSPARC Weather Station/Develop/VantagePro.dll" fn="_GetWindDir_V@0" ("Get Wind Dir")() -> ("return type"=w1217:i16)  [unwired: 3 in, 2 out]
                                n511 = To Single Precision Float(number=w1217) -> (single precision float=w1220:sgl)
                                n512 = call "Check_Value_Range.vi"("Min"=sgl 0.0, "Data in"=w1220, "Max"=sgl 360.0) -> ("Data out"=w1218:sgl)
                                n513 = call "Check_Data_Quality.vi"("Read sensor?"=w1219, "Data in"=w1218) -> ("Data out"=→"Cur wind dir":dbl)  [unwired: 1 out]
                                }
                                frame #2 {
                                n514 = call "Status_Error_Message.vi"("Message number"=239) -> ("Status/Error string"=w1222:string)
                                n515 = local write "Status/Error messages"(w1222) -> ()
                                }
                                }
                                }
                                }
                                }
                              }
                            }
                            frame #4 {
                              n516 = global read "Barometer_Calibration.vi" "Barometer sea level [hPa]"() -> (w1235:dbl)
                              n517 = global read "Barometer_Calibration.vi" "Station elevation [m]"() -> (w1234:i32)
                              n518 = Unbundle By Name(w1226) -> ("Path User Settings file"=w1225:path)
                              n519 = Not Equal?(x=w1235, y="Barometer sea level [hPa]") -> (x != y?=w1231:bool)
                              n520 = Not Equal?(x=w1234, y="Elevation [m]") -> (x != y?=w1230:bool)
                              n521 = Or(x=w1231, y=w1230) -> (x .or. y?=w1233:bool)
                              n522 = And(x=w1232, y=w1233) -> (x .and. y?=w1229:bool)
                              n523 = case shown="True" w1229 {
                                tunnel: w1225 -> [_ w1241]
                                tunnel: "Barometer sea level [hPa]" -> [_ w1242]
                                tunnel: "Elevation [m]" -> [_ w1239]
                                tunnel: [TRUE ("Calibration values set?") w1240] -> w1224
                                frame False {
                                n524 = call "Status_Error_Message.vi"("Message number"=140) -> ("Status/Error string"=w1236:string)
                                n525 = local write "Status/Error messages"(w1236) -> ()
                                }
                                frame True {
                                n526 = call "Set_Barometer_Calibration.vi"("Elevation"=w1239, "Sea level in"=w1242, "Path"=w1241) -> ("Calibration values set?"=w1240:bool)  [unwired: 1 out]
                                n527 = case shown="True" w1240 {
                                frame False {
                                n528 = call "Status_Error_Message.vi"("Message number"=340) -> ("Status/Error string"=w1244:string)
                                n529 = local write "Status/Error messages"(w1244) -> ()
                                }
                                frame True {
                                n530 = call "Status_Error_Message.vi"("Message number"=240) -> ("Status/Error string"=w1245:string)
                                n531 = local write "Status/Error messages"(w1245) -> ()
                                }
                                }
                                n532 = global write "Barometer_Calibration.vi" "Station elevation [m]"(w1239) -> ()
                                }
                              }
                            }
                            frame #5 {
                              n533 = Compound Arithmetic op=AND(w1250, w1251, w1249, w1247) -> (w1248:bool)
                              n534 = case shown="True" w1248 {
                                tunnel: ["Stop" ("y") "Read Weather Data" ("y")] -> w1252
                                frame False {
                                }
                                frame True {
                                w1255 = TRUE ("Visible")
                                # "Calibrationok or ignored, CONTINUE."
                                n535 = property on="Tab Control" class="TabCtl (strict)"("Visible"=w1255) -> ()  [unwired: 2 in, 2 out]
                                n536 = property on="Stop program?" class="Bool (strict)"("Visible"=w1255) -> ()  [unwired: 2 in, 2 out]
                                n537 = property on="DAQ software version" class="Str"("Visible"=w1255) -> ()  [unwired: 2 in, 2 out]
                                n538 = property on="DAQ mode?" class="Bool (strict)"("Visible"=w1255) -> ()  [unwired: 2 in, 2 out]
                                n539 = property on="Help?" class="Bool (strict)"("Visible"=w1255) -> ()  [unwired: 2 in, 2 out]
                                }
                              }
                            }
                          }
                        }
                      }
                    }
                    frame True {
                      # "'SAVE SETTINGS'."
                      n540 = Unbundle By Name(w1257) -> ("Path User Settings file"=w1256:path)
                      n541 = stacked-sequence {
                        seq-local: [w1263 _ _] -> [_ w1298 _]
                        tunnel: w1256 -> [w1294 _ _]
                        frame #0 {
                          w1268 = "Weather" ("key")
                          n542 = call <vilib>:"Open Config Data.vi"("create file if necessary (T)"=FALSE, "configuration file path"=w1294) -> ("refnum"=w1293:T4)  [unwired: 7 in, 2 out]
                          n543 = call-poly <vilib>:"Write Key.vi"("section"=w1268, "value"="Temperature inside", "key"="temperature_inside", "refnum"=w1293) -> ("refnum out"=w1278:T4)  [unwired: 5 in, 2 out]
                          n544 = call-poly <vilib>:"Write Key.vi"("section"=w1268, "value"="Temperature outside", "key"="temperature_outside", "refnum"=w1278) -> ("refnum out"=w1277:T4)  [unwired: 5 in, 2 out]
                          n545 = call-poly <vilib>:"Write Key.vi"("section"=w1268, "value"="Humidity inside", "key"="humidity_inside", "refnum"=w1277) -> ("refnum out"=w1276:T4)  [unwired: 5 in, 2 out]
                          n546 = call-poly <vilib>:"Write Key.vi"("section"=w1268, "value"="Wind speed", "key"="wind_speed", "refnum"=w1276) -> ("refnum out"=w1275:T4)  [unwired: 5 in, 2 out]
                          n547 = call-poly <vilib>:"Write Key.vi"("section"=w1268, "value"="Wind direction", "key"="wind_direction", "refnum"=w1275) -> ("refnum out"=w1274:T4)  [unwired: 5 in, 2 out]
                          n548 = call-poly <vilib>:"Write Key.vi"("section"=w1268, "value"="Barometer", "key"="barometer", "refnum"=w1274) -> ("refnum out"=w1273:T4)  [unwired: 5 in, 2 out]
                          n549 = call-poly <vilib>:"Write Key.vi"("section"=w1268, "value"="Humidity outside", "key"="humidity_outside", "refnum"=w1273) -> ("refnum out"=w1267:T4)  [unwired: 5 in, 2 out]
                          n550 = call-poly <vilib>:"Write Key.vi"("section"=w1268, "value"="Solar radiation", "key"="solar_radiation", "refnum"=w1267) -> ("refnum out"=w1266:T4)  [unwired: 5 in, 2 out]
                          n551 = call-poly <vilib>:"Write Key.vi"("section"=w1268, "value"="UV index", "key"="UV_index", "refnum"=w1266) -> ("refnum out"=w1265:T4)  [unwired: 5 in, 2 out]
                          n552 = call-poly <vilib>:"Write Key.vi"("section"=w1268, "value"="Evapotransipration rate", "key"="evapotranspiration", "refnum"=w1265) -> ("refnum out"=w1264:T4)  [unwired: 5 in, 2 out]
                          n553 = call-poly <vilib>:"Write Key.vi"("section"=w1268, "value"="Rain rate", "key"="rain_rate", "refnum"=w1264) -> ("refnum out"=w1263:T4)  [unwired: 5 in, 2 out]
                        }
                        frame #1 {
                          w1303 = "Weather" ("key")
                          n554 = call-poly <vilib>:"Write Key.vi"("section"=w1303, "value"="Wind chill", "key"="wind_chill", "refnum"=w1298) -> ("refnum out"=w1304:T4)  [unwired: 5 in, 2 out]
                          n555 = call-poly <vilib>:"Write Key.vi"("section"=w1303, "value"="Dew point", "key"="dew_point", "refnum"=w1304) -> ("refnum out"=w1312:T4)  [unwired: 5 in, 2 out]
                          n556 = call-poly <vilib>:"Write Key.vi"("section"=w1303, "value"="Heat index", "key"="heat_index", "refnum"=w1312) -> ("refnum out"=w1297:T4)  [unwired: 5 in, 2 out]
                          n557 = call-poly <vilib>:"Write Key.vi"("section"=w1303, "value"="Start in DAQ mode?", "key"="daq_mode", "refnum"=w1297) -> ("refnum out"=w1296:T4)  [unwired: 5 in, 2 out]
                          n558 = call-poly <vilib>:"Write Key.vi"("section"=w1303, "value"="Station ID", "key"="Station_ID", "refnum"=w1296) -> ("refnum out"=w1309:T4)  [unwired: 5 in, 2 out]
                          n559 = call-poly <vilib>:"Write Key.vi"("section"=w1303, "value"="Database name", "key"="Database_name", "refnum"=w1309) -> ("error out"=w1300:errorcluster, "refnum out"=w1299:T4)  [unwired: 5 in, 1 out]
                          n560 = call <vilib>:"Close Config Data.vi"("error in (no error)"=w1300, "refnum"=w1299) -> ()  [unwired: 8 in, 2 out]
                        }
                        frame #2 {
                          # "Keys have been saved"
                          n561 = call "Status_Error_Message.vi"("Message number"=125) -> ("Status/Error string"=w1318:string)
                          n562 = local write "Save settings?"(FALSE ("I have writen.")) -> ()
                          n563 = local write "Status/Error messages"(w1318) -> ()
                        }
                      }
                    }
                  }
                }
                frame True {
                  # "Stop execution!"
                  n564 = call "Status_Error_Message.vi"("Message number"=124) -> ("Status/Error string"=w1321:string)
                  n565 = local write "Status/Error messages"(w1321) -> ()
                }
              }
            }
            frame True {
              # "User pressed 'DAQ MODE' button."
              n566 = global read "DAQ_Mode.vi" "DAQ mode?"() -> (w1324:bool)
              n567 = case shown="False" w1324 {
                frame False {
                  w1328 = FALSE ("Visible")
                  # "Hide all buttons except the 'Stop DAQ' button"
                  n568 = property on="Tab Control" class="TabCtl (strict)"() -> ("Pages"=w1332:refnum<vi>[])  [unwired: 2 in, 2 out]
                  n569 = for {
                    tunnel: w1332 -> [w1334] mode=indexing
                    tunnel: bool[] [TRUE, TRUE, TRUE, TRUE, FALSE] -> [w1333] mode=indexing
                    n570 = property class="Page"(reference=w1334, "PageVis"=w1333) -> ()  [unwired: 1 in, 2 out]
                  }
                  n571 = property on="Stop program?" class="Bool (strict)"("Visible"=w1328) -> ()  [unwired: 2 in, 2 out]
                  n572 = property on="Help?" class="Bool (strict)"("Visible"=w1328) -> ()  [unwired: 2 in, 2 out]
                  n573 = call "Status_Error_Message.vi"("Message number"=123) -> ("Status/Error string"=w1330:string)
                  n574 = global write "DAQ_Mode.vi" "DAQ mode?"(TRUE ("DAQ mode?")) -> ()
                  n575 = local write "Status/Error messages"(w1330) -> ()
                }
                frame True {
                  # "Do nothing as the DAQ transfers\ndata to the buffer"
                }
              }
            }
          }
          n576 = global read "Stop_Data_Loop.vi" "Stop data loop"() -> (w1007:bool)
          n577 = Not Equal?(x=w1008, y="Read Weather Data") -> (x != y?=w1006:bool)
          n578 = Or(x=w1006, y=w1007) -> (x .or. y?=w1005:bool)
          n579 = global write "Stop_Button_Loop.vi" "Stop button loop"(w1005) -> ()
          n580 = Wait (ms)(milliseconds to wait=u32 50 ("millisecond multiple")) -> ()  [unwired: 1 out]
        }
        n581 = To Double Precision Float(number=w533) -> (double precision float=w532:dbl)
        n582 = Increment(x=w532) -> (x+1=w531:dbl)
        n583 = while {
          stop <- w975 stop-if-true
          n584 = global read "DAQ_Mode.vi" "DAQ mode?"() -> (w978:bool)
          n585 = Wait (ms)(milliseconds to wait=u32 1000 ("millisecond multiple")) -> ()  [unwired: 1 out]
          n586 = case shown="True" w978 {
            selector: w978 -> [w979 _]
            tunnel: [w979 w988] -> w977
            frame False {
              # "Not sending data to database"
            }
            frame True {
              w987 = FALSE ("create if not found? (T)")
              n587 = Obtain Queue(name (unnamed)="Database queue", element data type="" ("name (unnamed)"), create if not found? (T)=w987) -> (queue out=w985:refnum<queue>, error out=w986:errorcluster)  [unwired: 2 in, 1 out]
              n588 = Get Queue Status(queue=w985, return elements? (F)=w987, error in (no error)=w986) -> (queue out=w981:refnum<queue>, error out=w980:errorcluster, # elements in queue=w982:i32)  [unwired: 5 out]
              n589 = case shown="0" w982 {
                tunnel: [w989 w998] -> w988
                tunnel: w981 -> [_ w993]
                tunnel: w980 -> [_ w992]
                frame 0 {
                  # "No events to ship..."
                  n590 = local read "Buffer connected?"() -> (w989:bool)
                }
                frame 1, Default {
                  n591 = Dequeue Element(queue=w993, error in (no error)=w992) -> (element=w991:string, error out=w990:errorcluster)  [unwired: 1 in, 2 out]
                  n592 = local read "Database name"() -> (w995:string)
                  n593 = local read "Station ID"() -> (w994:i32)
                  n594 = call "Write_to_Database.vi"("Error in"=w990, "Database Name"=w995, "Weather Parameter String"=w991, "Detector ID"=w994) -> ("Error out"=w997:errorcluster, "Data Buffer?"=w996:bool)  [unwired: 2 in]
                  n595 = case shown="No Error" w997 {
                    tunnel: [w999 w1001] -> w998
                    tunnel: w996 -> [w999 w1001]
                    frame No Error {
                      # "Sending event to database"
                    }
                    frame Error {
                      n596 = call "Status_Error_Message.vi"("Message number"=323) -> ("Status/Error string"=w1003:string)
                      n597 = local write "Status/Error messages"(w1003) -> ()
                      n598 = local write "DAQ mode?"(FALSE ("DAQ mode?")) -> ()
                    }
                  }
                }
              }
            }
          }
          "Buffer connected?" <- w977
          n599 = global read "Stop_Data_Loop.vi" "Stop data loop"() -> (w975:bool)
        }
        n600 = while {
          tunnel: [w547] -> w536
          shift-right: [w542] -> _
          shift-left: w532 -> [w540]
          stop <- w549 stop-if-true
          # "Read data every 5 s"
          n601 = Get Date/Time In Seconds() -> (seconds since 1Jan1904=w546:timestamp)
          n602 = To Double Precision Float(number=w546) -> (double precision float=w543:dbl)
          n603 = Subtract(x=w543, y=w540) -> (x-y=w544:dbl)
          n604 = Greater Or Equal?(x=w544, y=5.0) -> (x >= y?=w541:bool)
          n605 = case shown="True" w541 {
            tunnel: ["Read Weather Data" w555] -> w547
            frame False {
              # "Wait for timer: read data once every 5 seconds..."
              n606 = Wait (ms)(milliseconds to wait=u32 100 ("millisecond multiple")) -> ()  [unwired: 1 out]
            }
            frame True {
              # "Weather data is loaded from the Vantage (Pro)\nconsole. If this failes, Labview tries 5 times\nbefore it closes the COM port and re-tries\n'Connect Weather Station'."
              n607 = while {
                tunnel: [w774] -> w556
                tunnel: [w778] -> w554
                i -> [w777]
                stop <- w779 stop-if-true
                n608 = dll-call lib="C:/Users/SuperUser/Desktop/HiSPARC Weather Station/Develop/VantagePro.dll" fn="_LoadCurrentVantageData_V@0" label="LoadCurrentVantageData"() -> ("return type"=w773:i16)  [unwired: 3 in, 2 out]
                n609 = Equal To 0?(x=w773) -> (x = 0?=w772:bool)
                n610 = case shown="True" w772 {
                  tunnel: [w781 w784] -> w778
                  tunnel: [FALSE TRUE] -> w774
                  frame False {
                    n611 = global read "PCtime_Last_Data.vi" "PC time last data"() -> (w781:timestamp)
                    n612 = Wait (ms)(milliseconds to wait=u32 100) -> ()  [unwired: 1 out]
                  }
                  frame True {
                    # "Timestamp"
                    n613 = Get Date/Time In Seconds() -> (seconds since 1Jan1904=w784:timestamp)
                  }
                }
                n614 = Less Or Equal?(x=5 ("y"), y=w777) -> (x <= y?=w775:bool)
                n615 = Or(x=w774, y=w775) -> (x .or. y?=w779:bool)
              }
              n616 = local write "Weather station connected?"(w556) -> ()
              n617 = global write "PCtime_Last_Data.vi" "PC time last data"(w554) -> ()
              n618 = case shown="True" w556 {
                tunnel: w554 -> [_ w628]
                tunnel: ["Connect Weather Station" "Read Weather Data"] -> w555
                frame False {
                  w583 = u32 6618880
                  w584 = u32 16711680
                  # "Run-time error!"
                  # "Failed to get data from weather station; try to:\n- Close port\n- Re-connect to weather station without user dialogue\n- All sensors offline"
                  n619 = flat-sequence {
                    frame #0 {
                      n620 = call "Status_Error_Message.vi"("Message number"=322) -> ("Status/Error string"=w604:string)
                      n621 = local write "Status/Error messages"(w604) -> ()
                    }
                    frame #1 {
                      # "Close connection"
                      n622 = call "Close_WeatherStation_Connection.vi"() -> ("Status/Error string"=w605:string)
                      n623 = local write "Status/Error messages"(w605) -> ()
                    }
                  }
                  n624 = local write "Run-time error"(TRUE ("Run-time error")) -> ()
                  n625 = local read "Evapotranspiration"() -> (w560:u32)
                  n626 = local read "Solar radiation"() -> (w563:u32)
                  n627 = local read "Wind direction"() -> (w565:u32)
                  n628 = local read "Temperature"() -> (w598:u32)
                  n629 = local read "Temperature"() -> (w581:u32)
                  n630 = local read "Wind speed"() -> (w564:u32)
                  n631 = local read "Heat index"() -> (w559:u32)
                  n632 = local read "Barometer"() -> (w566:u32)
                  n633 = local read "Dew point"() -> (w558:u32)
                  n634 = local read "Wind chill"() -> (w557:u32)
                  n635 = local read "UV index"() -> (w562:u32)
                  n636 = local read "Humidity"() -> (w579:u32)
                  n637 = local read "Humidity"() -> (w577:u32)
                  n638 = local read "Rain"() -> (w561:u32)
                  n639 = Equal?(x=w598, y=w583) -> (x = y?=w600:bool)
                  n640 = Equal?(x=w581, y=w583) -> (x = y?=w597:bool)
                  n641 = Equal?(x=w579, y=w583) -> (x = y?=w596:bool)
                  n642 = Equal?(x=w577, y=w583) -> (x = y?=w595:bool)
                  n643 = Equal?(x=w566, y=w583) -> (x = y?=w594:bool)
                  n644 = Equal?(x=w565, y=w583) -> (x = y?=w593:bool)
                  n645 = Equal?(x=w564, y=w583) -> (x = y?=w592:bool)
                  n646 = Equal?(x=w563, y=w583) -> (x = y?=w591:bool)
                  n647 = Equal?(x=w562, y=w583) -> (x = y?=w590:bool)
                  n648 = Equal?(x=w561, y=w583) -> (x = y?=w589:bool)
                  n649 = Equal?(x=w560, y=w583) -> (x = y?=w588:bool)
                  n650 = Equal?(x=w559, y=w583) -> (x = y?=w585:bool)
                  n651 = Equal?(x=w558, y=w583) -> (x = y?=w586:bool)
                  n652 = Equal?(x=w557, y=w583) -> (x = y?=w587:bool)
                  n653 = Select(t=w584, s=w600, f=w598) -> (s? t:f=w599:u32)
                  n654 = Select(t=w584, s=w597, f=w581) -> (s? t:f=w582:u32)
                  n655 = Select(t=w584, s=w596, f=w579) -> (s? t:f=w580:u32)
                  n656 = Select(t=w584, s=w595, f=w577) -> (s? t:f=w578:u32)
                  n657 = Select(t=w584, s=w594, f=w566) -> (s? t:f=w576:u32)
                  n658 = Select(t=w584, s=w593, f=w565) -> (s? t:f=w575:u32)
                  n659 = Select(t=w584, s=w592, f=w564) -> (s? t:f=w574:u32)
                  n660 = Select(t=w584, s=w591, f=w563) -> (s? t:f=w573:u32)
                  n661 = Select(t=w584, s=w590, f=w562) -> (s? t:f=w572:u32)
                  n662 = Select(t=w584, s=w589, f=w561) -> (s? t:f=w571:u32)
                  n663 = Select(t=w584, s=w588, f=w560) -> (s? t:f=w570:u32)
                  n664 = Select(t=w584, s=w585, f=w559) -> (s? t:f=w569:u32)
                  n665 = Select(t=w584, s=w586, f=w558) -> (s? t:f=w568:u32)
                  n666 = Select(t=w584, s=w587, f=w557) -> (s? t:f=w567:u32)
                  n667 = local write "Temperature"(w599) -> ()
                  n668 = local write "Temperature"(w582) -> ()
                  n669 = local write "Humidity"(w580) -> ()
                  n670 = local write "Humidity"(w578) -> ()
                  n671 = local write "Barometer"(w576) -> ()
                  n672 = local write "Wind direction"(w575) -> ()
                  n673 = local write "Wind speed"(w574) -> ()
                  n674 = local write "Solar radiation"(w573) -> ()
                  n675 = local write "UV index"(w572) -> ()
                  n676 = local write "Rain"(w571) -> ()
                  n677 = local write "Evapotranspiration"(w570) -> ()
                  n678 = local write "Heat index"(w569) -> ()
                  n679 = local write "Dew point"(w568) -> ()
                  n680 = local write "Wind chill"(w567) -> ()
                }
                frame True {
                  w626 = T3 {"Data out"=0.0, "Data out"=0.0, "Data out"=0.0, "Data out"=0.0, "Data out"=0.0, "Data out"=0.0, "Data out"=0.0, "Data out"=0.0, "Data out"=0.0, "Data out"=0.0, "Data out"=0.0, "Data out"=0.0, "Data out"=0.0, "Data out"=0.0, "seconds since 1Jan1904"=0.0} ("output cluster")
                  # "Any new measurements including\npc time stamp are added\nto the queue for histogramming"
                  n681 = local read "GPS time correction"() -> (w633:i32)
                  n682 = call "Read_Weather_Parameters.vi"("GPS time difference"=w633, "Current PC time"=w628) -> ("Weather data"=w634:T6, "Queue overflow?"=w618:bool, "Current GPS time"=→"GPS time last data":timestamp)  [unwired: 1 in]
                  n683 = case shown="True" w618 {
                    frame False {
                    }
                    frame True {
                      n684 = call "Status_Error_Message.vi"("Message number"=223) -> ("Status/Error string"=w770:string)
                      n685 = local write "Status/Error messages"(w770) -> ()
                    }
                  }
                  n686 = To Double Precision Float(number=w628) -> (double precision float=w627:dbl)
                  n687 = Unbundle By Name(w634) -> ("Temperature_inside"=w649:sgl, "Temperature_outside"=w650:sgl, "Humidity_inside"=w651:sgl, "Humidity_outside"=w652:sgl, "Barometer"=w653:sgl, "Wind_direction"=w654:sgl, "Wind_speed"=w655:sgl, "Solar_radiation"=w656:sgl, "UV_index"=w657:sgl, "Evapotranspiration"=w658:sgl, "Rain_rate"=w662:sgl, "Heat_index"=w659:sgl, "Dew_point"=w660:sgl, "Wind_chill"=w661:sgl)
                  n688 = local read "Evapotransipration rate"() -> (w672:bool)
                  n689 = local read "Temperature outside"() -> (w664:bool)
                  n690 = local read "Temperature inside"() -> (w663:bool)
                  n691 = local read "Humidity outside"() -> (w666:bool)
                  n692 = local read "Humidity inside"() -> (w665:bool)
                  n693 = local read "Solar radiation"() -> (w670:bool)
                  n694 = local read "Wind direction"() -> (w668:bool)
                  n695 = local read "Wind speed"() -> (w669:bool)
                  n696 = local read "Heat index"() -> (w674:bool)
                  n697 = local read "Barometer"() -> (w667:bool)
                  n698 = local read "Dew point"() -> (w675:bool)
                  n699 = local read "Rain rate"() -> (w673:bool)
                  n700 = local read "Wind chill"() -> (w676:bool)
                  n701 = local read "UV index"() -> (w671:bool)
                  n702 = call "Check_Data_Quality.vi"("Read sensor?"=w663, "Data in"=w649) -> ("Display colour"=→"Temperature":u32, "Data out"=w606:dbl)
                  "Temp in [°C]" <- w606
                  n703 = call "Check_Data_Quality.vi"("Read sensor?"=w664, "Data in"=w650) -> ("Display colour"=→"Temperature":u32, "Data out"=w607:dbl)
                  "Temp out [°C]" <- w607
                  n704 = call "Check_Data_Quality.vi"("Read sensor?"=w665, "Data in"=w651) -> ("Display colour"=→"Humidity":u32, "Data out"=w609:dbl)
                  "Hum in [%]" <- w609
                  n705 = call "Check_Data_Quality.vi"("Read sensor?"=w666, "Data in"=w652) -> ("Display colour"=→"Humidity":u32, "Data out"=w608:dbl)
                  "Hum out [%]" <- w608
                  n706 = call "Check_Data_Quality.vi"("Read sensor?"=w667, "Data in"=w653) -> ("Display colour"=→"Barometer":u32, "Data out"=w610:dbl)
                  "Barometer [hPa]" <- w610
                  n707 = call "Check_Data_Quality.vi"("Read sensor?"=w668, "Data in"=w654) -> ("Display colour"=→"Wind direction":u32, "Data out"=w620:dbl)
                  n708 = call "Check_Data_Quality.vi"("Read sensor?"=w669, "Data in"=w655) -> ("Display colour"=→"Wind speed":u32, "Data out"=w611:dbl)
                  "Wind speed [m/s]" <- w611
                  n709 = call "Check_Data_Quality.vi"("Read sensor?"=w670, "Data in"=w656) -> ("Display colour"=→"Solar radiation":u32, "Data out"=w613:dbl)
                  "Solar radiation [W/m²]" <- w613
                  n710 = call "Check_Data_Quality.vi"("Read sensor?"=w671, "Data in"=w657) -> ("Display colour"=→"UV index":u32, "Data out"=w612:dbl)
                  "UV index" <- w612
                  n711 = call "Check_Data_Quality.vi"("Read sensor?"=w672, "Data in"=w658) -> ("Display colour"=→"Evapotranspiration":u32, "Data out"=w616:dbl)
                  "Evapotranspiration" <- w616
                  n712 = call "Check_Data_Quality.vi"("Read sensor?"=w673, "Data in"=w662) -> ("Display colour"=→"Rain":u32, "Data out"=w614:dbl)
                  "Rain rate" <- w614
                  n713 = call "Check_Data_Quality.vi"("Read sensor?"=w674, "Data in"=w659) -> ("Display colour"=→"Heat index":u32, "Data out"=w622:dbl)
                  "Heat index [°C]" <- w622
                  n714 = call "Check_Data_Quality.vi"("Read sensor?"=w675, "Data in"=w660) -> ("Display colour"=→"Dew point":u32, "Data out"=w617:dbl)
                  "Dew point" <- w617
                  n715 = call "Check_Data_Quality.vi"("Read sensor?"=w676, "Data in"=w661) -> ("Display colour"=→"Wind chill":u32, "Data out"=w615:dbl)
                  "Wind chill [°C]" <- w615
                  n716 = Divide(x=w620, y=45.0) -> (x/y=→"Wind direction [º]":dbl)
                  n717 = Bundle(cluster=w626, "Data out"=w606, "Data out"=w607, "Data out"=w609, "Data out"=w608, "Data out"=w610, "Data out"=w620, "Data out"=w611, "Data out"=w613, "Data out"=w612, "Data out"=w616, "Data out"=w614, "Data out"=w622, "Data out"=w617, "Data out"=w615, "seconds since 1Jan1904"=w627) -> (w630:T3)
                  n718 = Obtain Queue(name (unnamed)="Weather data (5 s)", element data type=w626, create if not found? (T)=FALSE) -> (queue out=w631:refnum<queue>)  [unwired: 2 in, 2 out]
                  n719 = Lossy Enqueue Element(queue=w631, element=w630) -> (overflow?=w624:bool)  [unwired: 1 in, 3 out]
                  n720 = stacked-sequence {
                    seq-local: [w677 _ _ _ _ _] -> [_ _ _ _ w765 w767]
                    tunnel: w606 -> [_ _ w682 _ _ _]
                    tunnel: w607 -> [_ _ _ w726 _ _]
                    tunnel: w608 -> [_ _ _ w727 _ _]
                    tunnel: w610 -> [_ _ w704 _ _ _]
                    tunnel: w611 -> [_ _ _ w725 _ _]
                    tunnel: w612 -> [_ _ _ w742 _ _]
                    tunnel: w613 -> [_ _ w697 _ _ _]
                    tunnel: w616 -> [_ _ w690 _ _ _]
                    tunnel: w614 -> [_ _ _ w735 _ _]
                    tunnel: w617 -> [_ _ w683 _ _ _]
                    tunnel: w615 -> [_ _ _ w728 _ _]
                    tunnel: w609 -> [_ _ w681 _ _ _]
                    frame #0 {
                      # "Avoid switching to panel\neach time a unit is updated"
                      n721 = control-ref of="This VI"() -> (w679:refnum<vi>)
                      n722 = property class="VI"(reference=w679) -> ("Panel"=w677:refnum<vi>)  [unwired: 1 in, 2 out]
                      n723 = property class="Pnl"(reference=w677, "DeferPanUpdts"=TRUE ("Defer Panel Updates")) -> ()  [unwired: 1 in, 2 out]
                    }
                    frame #1 {
                      n724 = Wait (ms)(milliseconds to wait=u32 50) -> ()  [unwired: 1 out]
                    }
                    frame #2 {
                      n725 = local write "Cur in temp"(w682) -> ()
                      n726 = local write "Cur in hum"(w681) -> ()
                      n727 = local read "Temp. in High"() -> (w717:dbl)
                      n728 = local read "Temp. in Low"() -> (w718:dbl)
                      n729 = local read "Hum. in High"() -> (w711:dbl)
                      n730 = local read "Hum. in Low"() -> (w712:dbl)
                      n731 = local read "Evap. High"() -> (w696:dbl)
                      n732 = local read "Evap. Low"() -> (w695:dbl)
                      n733 = local read "Solar High"() -> (w698:dbl)
                      n734 = local read "Solar Low"() -> (w699:dbl)
                      n735 = local read "Dew High"() -> (w684:dbl)
                      n736 = local read "Bar. High"() -> (w705:dbl)
                      n737 = local read "Dew Low"() -> (w685:dbl)
                      n738 = local read "Bar. Low"() -> (w706:dbl)
                      n739 = Less?(x=w718, y=w682) -> (x < y?=w721:bool)
                      n740 = Greater?(x=w717, y=w682) -> (0:w722:bool)
                      n741 = Less?(x=w712, y=w681) -> (x < y?=w714:bool)
                      n742 = Greater?(x=w711, y=w681) -> (0:w713:bool)
                      n743 = Less?(x=w706, y=w704) -> (x < y?=w708:bool)
                      n744 = Greater?(x=w705, y=w704) -> (0:w707:bool)
                      n745 = Less?(x=w699, y=w697) -> (x < y?=w701:bool)
                      n746 = Greater?(x=w698, y=w697) -> (0:w700:bool)
                      n747 = Less?(x=w695, y=w690) -> (x < y?=w692:bool)
                      n748 = Greater?(x=w696, y=w690) -> (0:w691:bool)
                      n749 = Less?(x=w685, y=w683) -> (x < y?=w687:bool)
                      n750 = Greater?(x=w684, y=w683) -> (0:w686:bool)
                      n751 = Select(t=w718, s=w721, f=w682) -> (s? t:f=→"Temp. in Low":dbl)
                      n752 = Select(t=w717, s=w722, f=w682) -> (s? t:f=→"Temp. in High":dbl)
                      n753 = Select(t=w712, s=w714, f=w681) -> (s? t:f=→"Hum. in Low":dbl)
                      n754 = Select(t=w711, s=w713, f=w681) -> (s? t:f=→"Hum. in High":dbl)
                      n755 = Select(t=w706, s=w708, f=w704) -> (s? t:f=→"Bar. Low":dbl)
                      n756 = Select(t=w705, s=w707, f=w704) -> (s? t:f=→"Bar. High":dbl)
                      n757 = Select(t=w699, s=w701, f=w697) -> (s? t:f=→"Solar Low":dbl)
                      n758 = Select(t=w698, s=w700, f=w697) -> (s? t:f=→"Solar High":dbl)
                      n759 = Select(t=w695, s=w692, f=w690) -> (s? t:f=→"Evap. Low":dbl)
                      n760 = Select(t=w696, s=w691, f=w690) -> (s? t:f=→"Evap. High":dbl)
                      n761 = Select(t=w685, s=w687, f=w683) -> (s? t:f=→"Dew Low":dbl)
                      n762 = Select(t=w684, s=w686, f=w683) -> (s? t:f=→"Dew High":dbl)
                      "Temp. in" <- w682
                      "Cur bar" <- w704
                      "Dew" <- w683
                    }
                    frame #3 {
                      n763 = local write "Cur out temp"(w726) -> ()
                      n764 = local write "Cur out hum"(w727) -> ()
                      n765 = local read "Temp. out High"() -> (w759:dbl)
                      n766 = local read "Temp. out Low"() -> (w761:dbl)
                      n767 = local read "Hum. out High"() -> (w754:dbl)
                      n768 = local read "Hum. out Low"() -> (w755:dbl)
                      n769 = local read "Wind High"() -> (w748:dbl)
                      n770 = local read "Wind Low"() -> (w749:dbl)
                      n771 = local read "Rain High"() -> (w739:dbl)
                      n772 = local read "Rain Low"() -> (w736:dbl)
                      n773 = local read "Chill High"() -> (w729:dbl)
                      n774 = local read "Chill Low"() -> (w730:dbl)
                      n775 = local read "UV High"() -> (w743:dbl)
                      n776 = local read "UV Low"() -> (w724:dbl)
                      n777 = Less?(x=w761, y=w726) -> (x < y?=w762:bool)
                      n778 = Greater?(x=w759, y=w726) -> (0:w760:bool)
                      n779 = Less?(x=w755, y=w727) -> (x < y?=w756:bool)
                      n780 = Greater?(x=w754, y=w727) -> (0:w723:bool)
                      n781 = Less?(x=w749, y=w725) -> (x < y?=w751:bool)
                      n782 = Greater?(x=w748, y=w725) -> (0:w750:bool)
                      n783 = Less?(x=w724, y=w742) -> (x < y?=w745:bool)
                      n784 = Greater?(x=w743, y=w742) -> (0:w744:bool)
                      n785 = Less?(x=w736, y=w735) -> (x < y?=w738:bool)
                      n786 = Greater?(x=w739, y=w735) -> (0:w737:bool)
                      n787 = Less?(x=w730, y=w728) -> (x < y?=w732:bool)
                      n788 = Greater?(x=w729, y=w728) -> (0:w731:bool)
                      n789 = Select(t=w761, s=w762, f=w726) -> (s? t:f=→"Temp. out Low":dbl)
                      n790 = Select(t=w759, s=w760, f=w726) -> (s? t:f=→"Temp. out High":dbl)
                      n791 = Select(t=w755, s=w756, f=w727) -> (s? t:f=→"Hum. out Low":dbl)
                      n792 = Select(t=w754, s=w723, f=w727) -> (s? t:f=→"Hum. out High":dbl)
                      n793 = Select(t=w749, s=w751, f=w725) -> (s? t:f=→"Wind Low":dbl)
                      n794 = Select(t=w748, s=w750, f=w725) -> (s? t:f=→"Wind High":dbl)
                      n795 = Select(t=w724, s=w745, f=w742) -> (s? t:f=→"UV Low":dbl)
                      n796 = Select(t=w743, s=w744, f=w742) -> (s? t:f=→"UV High":dbl)
                      n797 = Select(t=w736, s=w738, f=w735) -> (s? t:f=→"Rain Low":dbl)
                      n798 = Select(t=w739, s=w737, f=w735) -> (s? t:f=→"Rain High":dbl)
                      n799 = Select(t=w730, s=w732, f=w728) -> (s? t:f=→"Chill Low":dbl)
                      n800 = Select(t=w729, s=w731, f=w728) -> (s? t:f=→"Chill High":dbl)
                      "Temp. out" <- w726
                      "Chill" <- w728
                    }
                    frame #4 {
                      # "Update panel"
                      n801 = property class="Pnl"(reference=w765, "DeferPanUpdts"=FALSE ("Defer Panel Updates")) -> ()  [unwired: 1 in, 2 out]
                    }
                    frame #5 {
                      n802 = Close Reference(reference=w767) -> ()  [unwired: 1 in, 1 out]
                    }
                  }
                  n803 = case shown="True" w624 {
                    frame False {
                    }
                    frame True {
                      n804 = call "Status_Error_Message.vi"("Message number"=224) -> ("Status/Error string"=w768:string)
                      n805 = local write "Status/Error messages"(w768) -> ()
                    }
                  }
                }
              }
            }
          }
          n806 = Select(t=w543, s=w541, f=w540) -> (s? t:f=w542:dbl)
          n807 = global read "Stop_Button_Loop.vi" "Stop button loop"() -> (w548:bool)
          n808 = Not Equal?(x=w547, y="Read Weather Data") -> (x != y?=w550:bool)
          n809 = Or(x=w550, y=w548) -> (x .or. y?=w549:bool)
          n810 = global write "Stop_Data_Loop.vi" "Stop data loop"(w549) -> ()
        }
        n811 = while {
          shift-right: [w790] -> _
          shift-left: w531 -> [w795]
          shift-right: [w791] -> _
          shift-left: w531 -> [w792]
          tunnel: w530 -> [w789]
          stop <- w798 stop-if-true
          n812 = Get Date/Time In Seconds() -> (seconds since 1Jan1904=w788:timestamp)
          n813 = To Double Precision Float(number=w788) -> (double precision float=w785:dbl)
          n814 = Subtract(x=w785, y=w795) -> (x-y=w796:dbl)
          n815 = Subtract(x=w785, y=w792) -> (x-y=w793:dbl)
          n816 = Greater Or Equal?(x=w796, y=60.0) -> (x >= y?=w787:bool)
          n817 = Greater Or Equal?(x=w793, y=600.0) -> (x >= y?=w786:bool)
          n818 = Select(t=w785, s=w786, f=w792) -> (s? t:f=w791:dbl)
          n819 = case shown="True" w786 {
            tunnel: w789 -> [_ w878]
            tunnel: w785 -> [_ w877]
            frame False {
              n820 = Wait (ms)(milliseconds to wait=u32 50) -> ()  [unwired: 1 out]
            }
            frame True {
              n821 = stacked-sequence {
                tunnel: w878 -> [w880 _]
                tunnel: w877 -> [w879 _]
                frame #0 {
                  n822 = stacked-sequence {
                    tunnel: w879 -> [w881 _ _ _ _]
                    tunnel: w880 -> [_ _ _ w895 _]
                    frame #0 {
                      # "Calculate 10 minutes averages;\nstore averages in graph queues"
                      n823 = call "Calculate_10Minutes_Averages.vi"("Current time"=w881) -> ()
                    }
                    frame #1 {
                      n824 = Wait (ms)(milliseconds to wait=u32 50) -> ()  [unwired: 1 out]
                    }
                    frame #2 {
                      # "Forecast"
                      n825 = dll-call lib="C:/Users/SuperUser/Desktop/HiSPARC Weather Station/Develop/VantagePro.dll" fn="_GetCurrentDataStrByID_V@12"("id"=u32 12, "string"="", "bufferlength"=i16 100) -> ("string"=w884:string)  [unwired: 6 in, 2 out]
                      n826 = Concatenate Strings("  ", w884) -> ()  [unwired: 1 out]
                      n827 = local write "Forecast"("  Forecast requires 3 hrs of recent data" ("Forecast")) -> ()
                    }
                    frame #3 {
                      # "GPS time correction?"
                      n828 = Unbundle By Name(w895) -> ("Path Run Status file"=w894:path)
                      n829 = call <vilib>:"Open Config Data.vi"("create file if necessary (T)"=FALSE, "configuration file path"=w894) -> ("error out"=w893:errorcluster, "refnum"=w896:T4)  [unwired: 7 in, 1 out]
                      n830 = call-poly <vilib>:"Read Key.vi"("section"="HiSPARC", "error in (no error)"=w893, "key"="time_difference", "refnum"=w896) -> ("error out"=w891:errorcluster, "value"=w889:i32, "refnum out"=w890:T4)  [unwired: 4 in, 1 out]
                      n831 = local write "GPS time correction"(w889) -> ()
                      n832 = call <vilib>:"Close Config Data.vi"("error in (no error)"=w891, "write file if changed (T)"=FALSE, "refnum"=w890) -> ()  [unwired: 7 in, 2 out]
                    }
                    frame #4 {
                      n833 = Wait (ms)(milliseconds to wait=u32 50) -> ()  [unwired: 1 out]
                    }
                  }
                }
                frame #1 {
                  n834 = Obtain Queue(name (unnamed)="48 hours data queue", element data type=T3 {"Data out"=0.0, "Data out"=0.0, "Data out"=0.0, "Data out"=0.0, "Data out"=0.0, "Data out"=0.0, "Data out"=0.0, "Data out"=0.0, "Data out"=0.0, "Data out"=0.0, "Data out"=0.0, "Data out"=0.0, "Data out"=0.0, "Data out"=0.0, "seconds since 1Jan1904"=0.0} ("output cluster"), create if not found? (T)=FALSE) -> (queue out=w904:refnum<queue>, error out=w905:errorcluster)  [unwired: 2 in, 1 out]
                  n835 = Get Queue Status(queue=w904, return elements? (F)=TRUE, error in (no error)=w905) -> (# elements in queue=w909:i32, elements=w906:T7)  [unwired: 6 out]
                  n836 = Greater Or Equal?(x=w909, y=2) -> (x >= y?=w908:bool)
                  n837 = case shown="True" w908 {
                    tunnel: w906 -> [_ w913]
                    tunnel: w909 -> [_ w912]
                    frame False {
                      # "Not enough events to display, yet!"
                      n838 = Wait (ms)(milliseconds to wait=u32 50) -> ()  [unwired: 1 out]
                    }
                    frame True {
                      n839 = stacked-sequence {
                        seq-local: [w914 _ _ _ _] -> [_ _ w971 _ w974]
                        tunnel: w913 -> [_ w928 _ _ _]
                        tunnel: w912 -> [_ w927 _ _ _]
                        frame #0 {
                          # "Avoid switching to panels\neach time a graph is updated"
                          n840 = control-ref of="This VI"() -> (w916:refnum<vi>)
                          n841 = property class="VI"(reference=w916) -> ("Panel"=w914:refnum<vi>)  [unwired: 1 in, 2 out]
                          n842 = property class="Pnl"(reference=w914, "DeferPanUpdts"=TRUE ("Defer Panel Updates")) -> ()  [unwired: 1 in, 2 out]
                        }
                        frame #1 {
                          n843 = for {
                            N: w927 -> [_]
                            tunnel: w928 -> [w970]
                            tunnel: [w967] -> w936 mode=indexing
                            tunnel: [w966] -> w935 mode=indexing
                            tunnel: [w965] -> w934 mode=indexing
                            tunnel: [w964] -> w933 mode=indexing
                            tunnel: [w963] -> w932 mode=indexing
                            tunnel: [w962] -> w919 mode=indexing
                            tunnel: [w961] -> w920 mode=indexing
                            tunnel: [w960] -> w931 mode=indexing
                            tunnel: [w959] -> w930 mode=indexing
                            tunnel: [w958] -> w924 mode=indexing
                            tunnel: [w957] -> w923 mode=indexing
                            tunnel: [w956] -> w925 mode=indexing
                            tunnel: [w955] -> w929 mode=indexing
                            tunnel: [w954] -> w938 mode=indexing
                            tunnel: [w953] -> w937 mode=indexing
                            i -> [w969]
                            n844 = Index Array(array=w970, index=w969) -> (element=w968:T3)
                            n845 = Unbundle(w968) -> ("Data out"=w967:dbl, "Data out"=w966:dbl, "Data out"=w965:dbl, "Data out"=w964:dbl, "Data out"=w963:dbl, "Data out"=w962:dbl, "Data out"=w961:dbl, "Data out"=w960:dbl, "Data out"=w959:dbl, "Data out"=w958:dbl, "Data out"=w957:dbl, "Data out"=w956:dbl, "Data out"=w955:dbl, "Data out"=w954:dbl, "seconds since 1Jan1904"=w953:dbl)
                          }
                          n846 = Bundle(w937, w936) -> (w940:cluster{dbl[], dbl[]})  [unwired: 1 in]
                          n847 = Bundle(w937, w935) -> (w939:cluster{dbl[], dbl[]})  [unwired: 1 in]
                          n848 = Bundle(w937, w934) -> (w942:cluster{dbl[], dbl[]})  [unwired: 1 in]
                          n849 = Bundle(w937, w933) -> (w941:cluster{dbl[], dbl[]})  [unwired: 1 in]
                          n850 = Bundle(w937, w932) -> (→"Barometer (48h)":cluster{dbl[], dbl[]})  [unwired: 1 in]
                          n851 = Bundle(w937, w920) -> (w944:cluster{dbl[], dbl[]})  [unwired: 1 in]
                          n852 = Bundle(w937, w919) -> (w943:cluster{dbl[], dbl[]})  [unwired: 1 in]
                          n853 = Bundle(w937, w931) -> (→"Solar radiation (48h)":cluster{dbl[], dbl[]})  [unwired: 1 in]
                          n854 = Bundle(w937, w930) -> (→"UV (48h)":cluster{dbl[], dbl[]})  [unwired: 1 in]
                          n855 = Bundle(w937, w924) -> (w946:cluster{dbl[], dbl[]})  [unwired: 1 in]
                          n856 = Bundle(w937, w925) -> (w945:cluster{dbl[], dbl[]})  [unwired: 1 in]
                          n857 = Bundle(w937, w923) -> (w948:cluster{dbl[], dbl[]})  [unwired: 1 in]
                          n858 = Bundle(w937, w929) -> (w947:cluster{dbl[], dbl[]})  [unwired: 1 in]
                          n859 = Bundle(w937, w938) -> (→"Wind chill (48h)":cluster{dbl[], dbl[]})  [unwired: 1 in]
                          n860 = Build Array(w940, w939) -> (→"Temperatures (48h)":cluster{dbl[], dbl[]}[])
                          n861 = Build Array(w942, w941) -> (→"Humidities (48h)":cluster{dbl[], dbl[]}[])
                          n862 = Build Array(w944, w943) -> (→"Wind (48h)":cluster{dbl[], dbl[]}[])
                          n863 = Build Array(w946, w945) -> (→"Evap & heat (48h])":cluster{dbl[], dbl[]}[])
                          n864 = Build Array(w948, w947) -> (→"Rain & dew (48h)":cluster{dbl[], dbl[]}[])
                        }
                        frame #2 {
                          # "Update graphs"
                          n865 = property class="Pnl"(reference=w971, "DeferPanUpdts"=FALSE ("Defer Panel Updates")) -> ()  [unwired: 1 in, 2 out]
                        }
                        frame #3 {
                          n866 = Wait (ms)(milliseconds to wait=u32 20) -> ()  [unwired: 1 out]
                        }
                        frame #4 {
                          n867 = Close Reference(reference=w974) -> ()  [unwired: 1 in, 1 out]
                        }
                      }
                    }
                  }
                }
              }
            }
          }
          n868 = Select(t=w785, s=w787, f=w795) -> (s? t:f=w790:dbl)
          n869 = case shown="True" w787 {
            tunnel: w785 -> [_ w800]
            frame False {
              n870 = Wait (ms)(milliseconds to wait=u32 50) -> ()  [unwired: 1 out]
            }
            frame True {
              n871 = stacked-sequence {
                tunnel: w800 -> [w801 _]
                frame #0 {
                  # "Calculate 1 minute averages;\nstore averages in graph queues"
                  n872 = call "Calculate_1Minute_Averages.vi"("Current time"=w801) -> ()
                }
                frame #1 {
                  n873 = Obtain Queue(name (unnamed)="60 minutes data queue", element data type=T3 {"Data out"=0.0, "Data out"=0.0, "Data out"=0.0, "Data out"=0.0, "Data out"=0.0, "Data out"=0.0, "Data out"=0.0, "Data out"=0.0, "Data out"=0.0, "Data out"=0.0, "Data out"=0.0, "Data out"=0.0, "Data out"=0.0, "Data out"=0.0, "seconds since 1Jan1904"=0.0} ("output cluster"), create if not found? (T)=FALSE) -> (queue out=w806:refnum<queue>, error out=w807:errorcluster)  [unwired: 2 in, 1 out]
                  n874 = Get Queue Status(queue=w806, return elements? (F)=TRUE, error in (no error)=w807) -> (# elements in queue=w802:i32, elements=w803:T7)  [unwired: 6 out]
                  n875 = Greater Or Equal?(x=w802, y=2) -> (x >= y?=w810:bool)
                  n876 = case shown="True" w810 {
                    tunnel: w803 -> [_ w814]
                    tunnel: w802 -> [_ w813]
                    frame False {
                      # "Not enough events to display, yet!"
                      n877 = Wait (ms)(milliseconds to wait=u32 50) -> ()  [unwired: 1 out]
                    }
                    frame True {
                      n878 = stacked-sequence {
                        seq-local: [w815 _ _ _ _] -> [_ _ w872 _ w875]
                        tunnel: w814 -> [_ w839 _ _ _]
                        tunnel: w813 -> [_ w825 _ _ _]
                        frame #0 {
                          # "Avoid switching to panels\neach time a graph is updated"
                          n879 = control-ref of="This VI"() -> (w817:refnum<vi>)
                          n880 = property class="VI"(reference=w817) -> ("Panel"=w815:refnum<vi>)  [unwired: 1 in, 2 out]
                          n881 = property class="Pnl"(reference=w815, "DeferPanUpdts"=TRUE ("Defer Panel Updates")) -> ()  [unwired: 1 in, 2 out]
                        }
                        frame #1 {
                          n882 = for {
                            N: w825 -> [_]
                            tunnel: w839 -> [w871]
                            tunnel: [w868] -> w826 mode=indexing
                            tunnel: [w867] -> w827 mode=indexing
                            tunnel: [w866] -> w828 mode=indexing
                            tunnel: [w865] -> w829 mode=indexing
                            tunnel: [w864] -> w830 mode=indexing
                            tunnel: [w863] -> w838 mode=indexing
                            tunnel: [w862] -> w837 mode=indexing
                            tunnel: [w861] -> w836 mode=indexing
                            tunnel: [w860] -> w835 mode=indexing
                            tunnel: [w859] -> w831 mode=indexing
                            tunnel: [w858] -> w832 mode=indexing
                            tunnel: [w857] -> w833 mode=indexing
                            tunnel: [w856] -> w818 mode=indexing
                            tunnel: [w855] -> w819 mode=indexing
                            tunnel: [w854] -> w834 mode=indexing
                            i -> [w870]
                            n883 = Index Array(array=w871, index=w870) -> (element=w869:T3)
                            n884 = Unbundle(w869) -> ("Data out"=w868:dbl, "Data out"=w867:dbl, "Data out"=w866:dbl, "Data out"=w865:dbl, "Data out"=w864:dbl, "Data out"=w856:dbl, "Data out"=w855:dbl, "Data out"=w859:dbl, "Data out"=w858:dbl, "Data out"=w857:dbl, "Data out"=w854:dbl, "Data out"=w860:dbl, "Data out"=w861:dbl, "Data out"=w862:dbl, "seconds since 1Jan1904"=w863:dbl)
                          }
                          n885 = Bundle(w838, w826) -> (w852:cluster{dbl[], dbl[]})  [unwired: 1 in]
                          n886 = Bundle(w838, w827) -> (w853:cluster{dbl[], dbl[]})  [unwired: 1 in]
                          n887 = Bundle(w838, w828) -> (w849:cluster{dbl[], dbl[]})  [unwired: 1 in]
                          n888 = Bundle(w838, w829) -> (w850:cluster{dbl[], dbl[]})  [unwired: 1 in]
                          n889 = Bundle(w838, w830) -> (→"Barometer (1h)":cluster{dbl[], dbl[]})  [unwired: 1 in]
                          n890 = Bundle(w838, w819) -> (w845:cluster{dbl[], dbl[]})  [unwired: 1 in]
                          n891 = Bundle(w838, w818) -> (w846:cluster{dbl[], dbl[]})  [unwired: 1 in]
                          n892 = Bundle(w838, w831) -> (→"Solar radiation (1h)":cluster{dbl[], dbl[]})  [unwired: 1 in]
                          n893 = Bundle(w838, w832) -> (→"UV (1h)":cluster{dbl[], dbl[]})  [unwired: 1 in]
                          n894 = Bundle(w838, w833) -> (w843:cluster{dbl[], dbl[]})  [unwired: 1 in]
                          n895 = Bundle(w838, w835) -> (w844:cluster{dbl[], dbl[]})  [unwired: 1 in]
                          n896 = Bundle(w838, w834) -> (w841:cluster{dbl[], dbl[]})  [unwired: 1 in]
                          n897 = Bundle(w838, w836) -> (w842:cluster{dbl[], dbl[]})  [unwired: 1 in]
                          n898 = Bundle(w838, w837) -> (→"Wind chill (1h)":cluster{dbl[], dbl[]})  [unwired: 1 in]
                          n899 = Build Array(w852, w853) -> (→"Temperatures (1h)":cluster{dbl[], dbl[]}[])
                          n900 = Build Array(w849, w850) -> (→"Humidities (1h)":cluster{dbl[], dbl[]}[])
                          n901 = Build Array(w845, w846) -> (→"Wind (1h)":cluster{dbl[], dbl[]}[])
                          n902 = Build Array(w843, w844) -> (→"Evap & heat (1h])":cluster{dbl[], dbl[]}[])
                          n903 = Build Array(w841, w842) -> (→"Rain & dew (1h)":cluster{dbl[], dbl[]}[])
                        }
                        frame #2 {
                          # "Update graphs"
                          n904 = property class="Pnl"(reference=w872, "DeferPanUpdts"=FALSE ("Defer Panel Updates")) -> ()  [unwired: 1 in, 2 out]
                        }
                        frame #3 {
                          n905 = Wait (ms)(milliseconds to wait=u32 20) -> ()  [unwired: 1 out]
                        }
                        frame #4 {
                          n906 = Close Reference(reference=w875) -> ()  [unwired: 1 in, 1 out]
                        }
                      }
                    }
                  }
                }
              }
            }
          }
          n907 = global read "Stop_Data_Loop.vi" "Stop data loop"() -> (w798:bool)
        }
        n908 = Equal?(x="Read Weather Data" ("y"), y=w536) -> (x = y?=w537:bool)
        n909 = Select(t=w534, s=w537, f=w536) -> (s? t:f=w535:string)
      }
      frame "Stop" {
        n910 = flat-sequence {
          tunnel: w1338 -> [w1342]
          tunnel: [w1342] -> w1336
          tunnel: [w1347] -> w1337
          tunnel: w1336 -> [w1347]
          tunnel: [w1343] -> w1335
          frame #0 {
            w1341 = FALSE ("Visible")
            n911 = property on="Tab Control" class="TabCtl (strict)"("Visible"=w1341) -> ()  [unwired: 2 in, 2 out]
            n912 = property on="Stop program?" class="Bool (strict)"("Visible"=w1341) -> ()  [unwired: 2 in, 2 out]
            n913 = property on="DAQ mode?" class="Bool (strict)"("Visible"=w1341) -> ()  [unwired: 2 in, 2 out]
            n914 = property on="Help?" class="Bool (strict)"("Visible"=w1341) -> ()  [unwired: 2 in, 2 out]
            n915 = property on="DAQ software version" class="Str"("Visible"=w1341) -> ()  [unwired: 2 in, 2 out]
          }
          frame #1 {
            n916 = Two Button Dialog(message="Do you realy wish to quit?", 1:"NO" ("F button name (\"Cancel\")"), 2:"YES" ("T button name (\"OK\")")) -> (T button?=w1343:bool)
          }
        }
        n917 = case shown="True" w1335 {
          tunnel: [w1348 w1369] -> w1339
          tunnel: w1337 -> [_ w1370]
          frame False {
            n918 = local write "Stop program?"(FALSE ("Stop program?")) -> ()
            n919 = Two Button Dialog(message="Do you wish to re-initialise the DAQ program?\n(settings will be read from user initialisation file and graphs will be cleared!)", 1:"NO" ("F button name (\"Cancel\")"), 2:"YES" ("T button name (\"OK\")")) -> (T button?=w1351:bool)
            n920 = case shown="False" w1351 {
              tunnel: ["Read Weather Data" ("y") "Initialise" ("y")] -> w1349
              frame False {
                w1357 = FALSE
                (unwired) "Stop weather station ignored, CONTINUE." ("string")
                # "Stop conditions while taking data"
                n921 = global write "Stop_Button_Loop.vi" "Stop button loop"(w1357) -> ()
                n922 = global write "Stop_Data_Loop.vi" "Stop data loop"(w1357) -> ()
                n923 = call "Status_Error_Message.vi"("Message number"=103) -> ("Status/Error string"=w1360:string)
                n924 = local write "Status/Error messages"(w1360) -> ()
              }
              frame True {
                n925 = stacked-sequence {
                  frame #0 {
                    n926 = call "Status_Error_Message.vi"("Message number"=3) -> ("Status/Error string"=w1362:string)
                    n927 = local write "Status/Error messages"(w1362) -> ()
                  }
                  frame #1 {
                    # "Close connection"
                    n928 = call "Close_WeatherStation_Connection.vi"() -> ("Status/Error string"=w1364:string)
                    n929 = local write "Status/Error messages"(w1364) -> ()
                  }
                }
              }
            }
            n930 = flat-sequence {
              tunnel: w1349 -> [w1356]
              tunnel: [w1356] -> w1348
              frame #0 {
                w1355 = TRUE ("Visible")
                n931 = property on="Tab Control" class="TabCtl (strict)"("Visible"=w1355) -> ()  [unwired: 2 in, 2 out]
                n932 = property on="Stop program?" class="Bool (strict)"("Visible"=w1355) -> ()  [unwired: 2 in, 2 out]
                n933 = property on="DAQ mode?" class="Bool (strict)"("Visible"=w1355) -> ()  [unwired: 2 in, 2 out]
                n934 = property on="Help?" class="Bool (strict)"("Visible"=w1355) -> ()  [unwired: 2 in, 2 out]
                n935 = property on="DAQ software version" class="Str"("Visible"=w1355) -> ()  [unwired: 2 in, 2 out]
              }
            }
          }
          frame True {
            n936 = flat-sequence {
              tunnel: w1370 -> [w1371]
              tunnel: [w1371] -> w1366
              tunnel: [w1393] -> w1367
              tunnel: w1366 -> [w1393]
              tunnel: [w1397] -> w1368
              tunnel: w1367 -> [w1397]
              tunnel: [w1412] -> w1365
              tunnel: w1368 -> [w1412]
              tunnel: [w1414] -> w1369
              tunnel: w1365 -> [w1414]
              frame #0 {
                n937 = stacked-sequence {
                  frame #0 {
                    n938 = Obtain Queue(name (unnamed)="Weather data (5 s)", element data type=T3 {"Data out"=0.0, "Data out"=0.0, "Data out"=0.0, "Data out"=0.0, "Data out"=0.0, "Data out"=0.0, "Data out"=0.0, "Data out"=0.0, "Data out"=0.0, "Data out"=0.0, "Data out"=0.0, "Data out"=0.0, "Data out"=0.0, "Data out"=0.0, "seconds since 1Jan1904"=0.0} ("output cluster"), create if not found? (T)=FALSE) -> (queue out=w1376:refnum<queue>, error out=w1373:errorcluster)  [unwired: 2 in, 1 out]
                    n939 = Obtain Queue(name (unnamed)="Database queue", element data type="" ("Weather parameter string"), create if not found? (T)=FALSE) -> (queue out=w1380:refnum<queue>, error out=w1372:errorcluster)  [unwired: 2 in, 1 out]
                    n940 = Flush Queue(queue=w1376, error in (no error)=w1373) -> ()  [unwired: 3 out]
                    n941 = Flush Queue(queue=w1380, error in (no error)=w1372) -> ()  [unwired: 3 out]
                  }
                  frame #1 {
                    n942 = Obtain Queue(name (unnamed)="60 minutes data queue", element data type=T3 {"Data out"=0.0, "Data out"=0.0, "Data out"=0.0, "Data out"=0.0, "Data out"=0.0, "Data out"=0.0, "Data out"=0.0, "Data out"=0.0, "Data out"=0.0, "Data out"=0.0, "Data out"=0.0, "Data out"=0.0, "Data out"=0.0, "Data out"=0.0, "seconds since 1Jan1904"=0.0} ("output cluster"), create if not found? (T)=FALSE) -> (queue out=w1390:refnum<queue>, error out=w1383:errorcluster)  [unwired: 2 in, 1 out]
                    n943 = Obtain Queue(name (unnamed)="48 hours data queue", element data type=T3 {"Data out"=0.0, "Data out"=0.0, "Data out"=0.0, "Data out"=0.0, "Data out"=0.0, "Data out"=0.0, "Data out"=0.0, "Data out"=0.0, "Data out"=0.0, "Data out"=0.0, "Data out"=0.0, "Data out"=0.0, "Data out"=0.0, "Data out"=0.0, "seconds since 1Jan1904"=0.0} ("output cluster"), create if not found? (T)=FALSE) -> (queue out=w1386:refnum<queue>, error out=w1382:errorcluster)  [unwired: 2 in, 1 out]
                    n944 = Flush Queue(queue=w1390, error in (no error)=w1383) -> ()  [unwired: 3 out]
                    n945 = Flush Queue(queue=w1386, error in (no error)=w1382) -> ()  [unwired: 3 out]
                  }
                  frame #2 {
                    # "Close connection"
                    n946 = call "Close_WeatherStation_Connection.vi"() -> ("Status/Error string"=w1392:string)
                    n947 = local write "Status/Error messages"(w1392) -> ()
                  }
                }
              }
              frame #1 {
                n948 = Wait (ms)(milliseconds to wait=u32 20) -> ()  [unwired: 1 out]
              }
              frame #2 {
                n949 = control-ref of="This VI"() -> (w1396:refnum<vi>)
                n950 = property class="VI"(reference=w1396) -> ("Panel"=w1395:refnum<vi>)  [unwired: 1 in, 2 out]
                n951 = stacked-sequence {
                  tunnel: w1395 -> [w1398 _ _ _ w1407 _ w1410]
                  frame #0 {
                    # "Re-initialise graphs"
                    # "Avoid switching to panels\neach time a unit is updated"
                    n952 = property class="Pnl"(reference=w1398, "DeferPanUpdts"=TRUE ("Defer Panel Updates")) -> ()  [unwired: 1 in, 2 out]
                  }
                  frame #1 {
                    n953 = invoke on="Temperatures (1h)" class="XYGraph (strict)" method="Reinit To Default"() -> ()  [unwired: 3 in, 3 out]
                    n954 = invoke on="Humidities (1h)" class="XYGraph (strict)" method="Reinit To Default"() -> ()  [unwired: 3 in, 3 out]
                    n955 = invoke on="Rain & dew (1h)" class="XYGraph (strict)" method="Reinit To Default"() -> ()  [unwired: 3 in, 3 out]
                    n956 = invoke on="Evap & heat (1h])" class="XYGraph (strict)" method="Reinit To Default"() -> ()  [unwired: 3 in, 3 out]
                    n957 = invoke on="Wind (1h)" class="XYGraph (strict)" method="Reinit To Default"() -> ()  [unwired: 3 in, 3 out]
                    n958 = invoke on="Barometer (1h)" class="XYGraph (strict)" method="Reinit To Default"() -> ()  [unwired: 3 in, 3 out]
                    n959 = invoke on="Wind chill (1h)" class="XYGraph (strict)" method="Reinit To Default"() -> ()  [unwired: 3 in, 3 out]
                    n960 = invoke on="Solar radiation (1h)" class="XYGraph (strict)" method="Reinit To Default"() -> ()  [unwired: 3 in, 3 out]
                    n961 = invoke on="UV (1h)" class="XYGraph (strict)" method="Reinit To Default"() -> ()  [unwired: 3 in, 3 out]
                  }
                  frame #2 {
                    n962 = invoke on="Temperatures (48h)" class="XYGraph (strict)" method="Reinit To Default"() -> ()  [unwired: 3 in, 3 out]
                    n963 = invoke on="Humidities (48h)" class="XYGraph (strict)" method="Reinit To Default"() -> ()  [unwired: 3 in, 3 out]
                    n964 = invoke on="Rain & dew (48h)" class="XYGraph (strict)" method="Reinit To Default"() -> ()  [unwired: 3 in, 3 out]
                    n965 = invoke on="Evap & heat (48h])" class="XYGraph (strict)" method="Reinit To Default"() -> ()  [unwired: 3 in, 3 out]
                    n966 = invoke on="Wind (48h)" class="XYGraph (strict)" method="Reinit To Default"() -> ()  [unwired: 3 in, 3 out]
                    n967 = invoke on="Barometer (48h)" class="XYGraph (strict)" method="Reinit To Default"() -> ()  [unwired: 3 in, 3 out]
                    n968 = invoke on="Wind chill (48h)" class="XYGraph (strict)" method="Reinit To Default"() -> ()  [unwired: 3 in, 3 out]
                    n969 = invoke on="Solar radiation (48h)" class="XYGraph (strict)" method="Reinit To Default"() -> ()  [unwired: 3 in, 3 out]
                    n970 = invoke on="UV (48h)" class="XYGraph (strict)" method="Reinit To Default"() -> ()  [unwired: 3 in, 3 out]
                  }
                  frame #3 {
                    w1402 = TRUE ("Visible")
                    # "Stop HiSPARC weather station DAQ"
                    n971 = property on="Tab Control" class="TabCtl (strict)"("Visible"=w1402) -> ()  [unwired: 2 in, 2 out]
                    n972 = call "Status_Error_Message.vi"("Message number"=2) -> ("Status/Error string"=w1404:string)
                    n973 = property on="Stop program?" class="Bool (strict)"("Visible"=w1402) -> ()  [unwired: 2 in, 2 out]
                    n974 = property on="DAQ software version" class="Str"("Visible"=w1402) -> ()  [unwired: 2 in, 2 out]
                    n975 = local write "Status/Error messages"(w1404) -> ()
                    n976 = property on="DAQ mode?" class="Bool (strict)"("Visible"=w1402) -> ()  [unwired: 2 in, 2 out]
                    n977 = property on="Help?" class="Bool (strict)"("Visible"=w1402) -> ()  [unwired: 2 in, 2 out]
                    n978 = property on="Tab Control" class="TabCtl (strict)"() -> ("Pages"=w1401:refnum<vi>[])  [unwired: 2 in, 2 out]
                    n979 = for {
                      tunnel: w1401 -> [w1406] mode=indexing
                      tunnel: bool[] [TRUE, TRUE, TRUE, TRUE, TRUE] -> [w1405] mode=indexing
                      n980 = property class="Page"(reference=w1406, "PageVis"=w1405) -> ()  [unwired: 1 in, 2 out]
                    }
                  }
                  frame #4 {
                    # "Update panels"
                    n981 = property class="Pnl"(reference=w1407, "DeferPanUpdts"=FALSE ("Defer Panel Updates")) -> ()  [unwired: 1 in, 2 out]
                  }
                  frame #5 {
                    n982 = Wait (ms)(milliseconds to wait=u32 20) -> ()  [unwired: 1 out]
                  }
                  frame #6 {
                    n983 = Close Reference(reference=w1410) -> ()  [unwired: 1 in, 1 out]
                  }
                }
              }
              frame #3 {
                n984 = local write "Stop program?"(FALSE ("Stop program?")) -> ()
              }
              frame #4 {
                n985 = Stop(stop? (T)=TRUE ("Visible")) -> ()
              }
            }
          }
        }
      }
    }
  }
